vi "Entrenamiento Fuerza temp.vi"(8 "error in (no error)":errorcluster) -> (0 "error out":errorcluster)   [LabVIEW 2014]
panel:
  out "element":T1
  in  "Master":bool
  out "OK":bool
  out "error out 2":errorcluster
  in  "Puerto Serial":refnum<visa-resource-name>="COM12"
  in  "index":i32
  out "size(s)":i32
  out "Decorations[]":refnum<vi>[](array[refnum])
  out "Boolean":bool
  in  "Start":bool
  in  "Impulso":bool
  in  "Reset":bool
  in  "Back":bool
  in  "Help":bool
  in  "Slider":i32(slide) scale=0.0..100.0
  in  "Remove Button":bool
  in  "Add Button":bool
  in  "Opcional Bool":bool
  in  "Biceps Bool":bool
  in  "Pectorales Bool":bool
  in  "Trapecio Bool":bool
  in  "Dorsales Bool":bool
  in  "Lumbares Bool":bool
  in  "Abdomen Bool":bool
  in  "Gluteos Bool":bool
  in  "Isquiotibiales Bool":bool
  in  "Stop":bool
  in  "Cuadriceps Bool":bool
  # "Entrenamiento de Fuerza"
  # "Presentación"
  # "Seg"
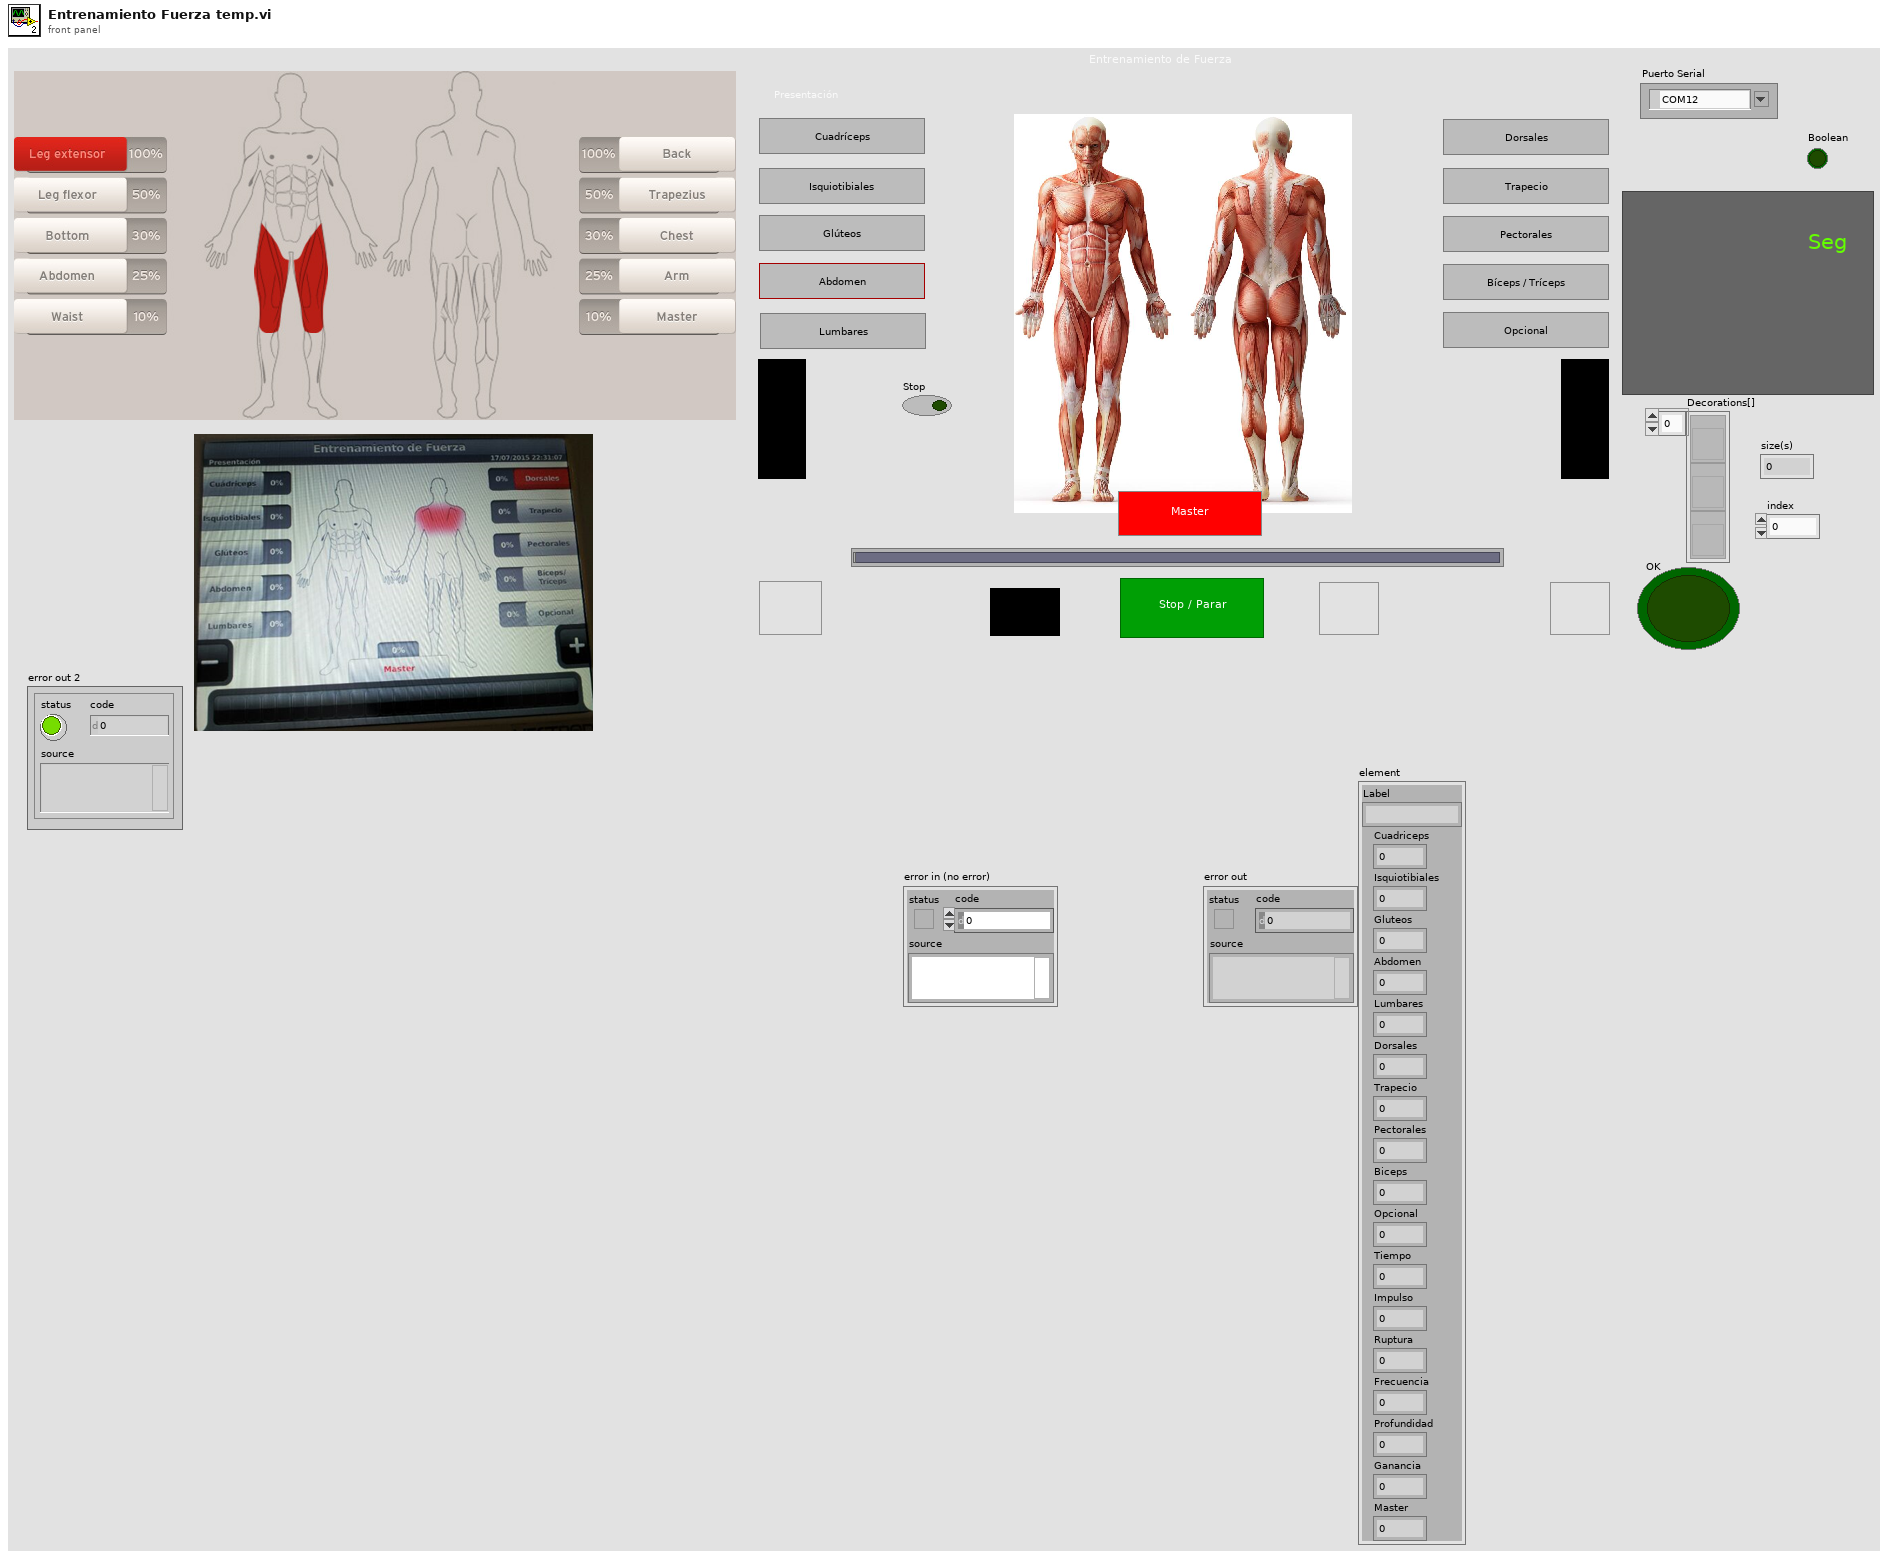
[diagram p1: front panel]
types:
  T1 = cluster{"Label":string, "Cuadriceps":i32, "Isquiotibiales":i32, "Gluteos":i32, "Abdomen":i32, "Lumbares":i32, "Dorsales":i32, "Trapecio":i32, "Pectorales":i32, "Biceps":i32, "Opcional":i32, "Tiempo":i32, "Impulso":i32, "Ruptura":i32, "Frecuencia":i32, "Profundidad":i32, "Ganancia":dbl, "Master":i32}
  T2 = cluster{"Boolean Text.Text Colors:Text Color":u32, u32}
  T3 = cluster{u32, "Boolean Text.Text Colors:Text Color":u32}
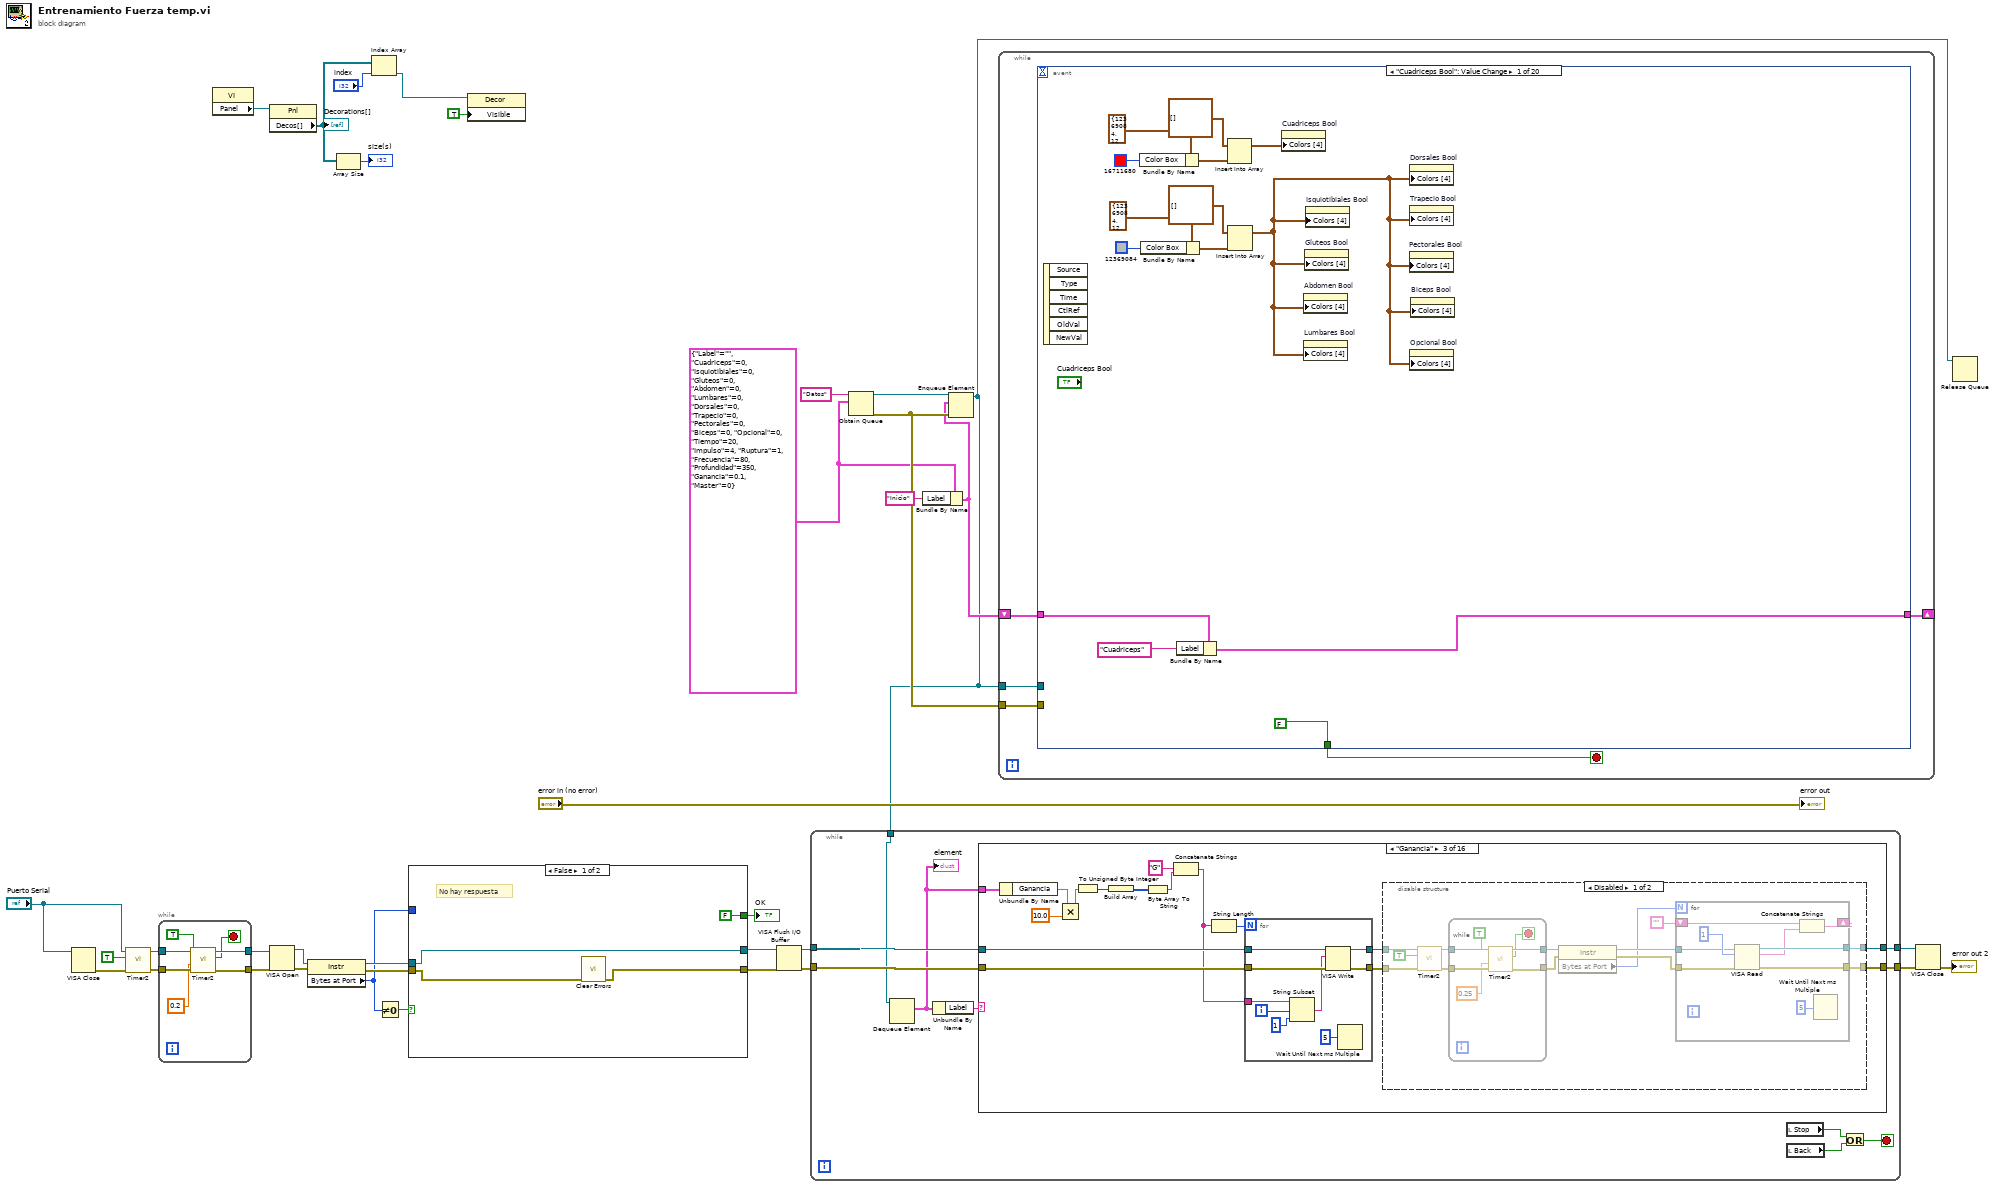
[diagram p0: block diagram]
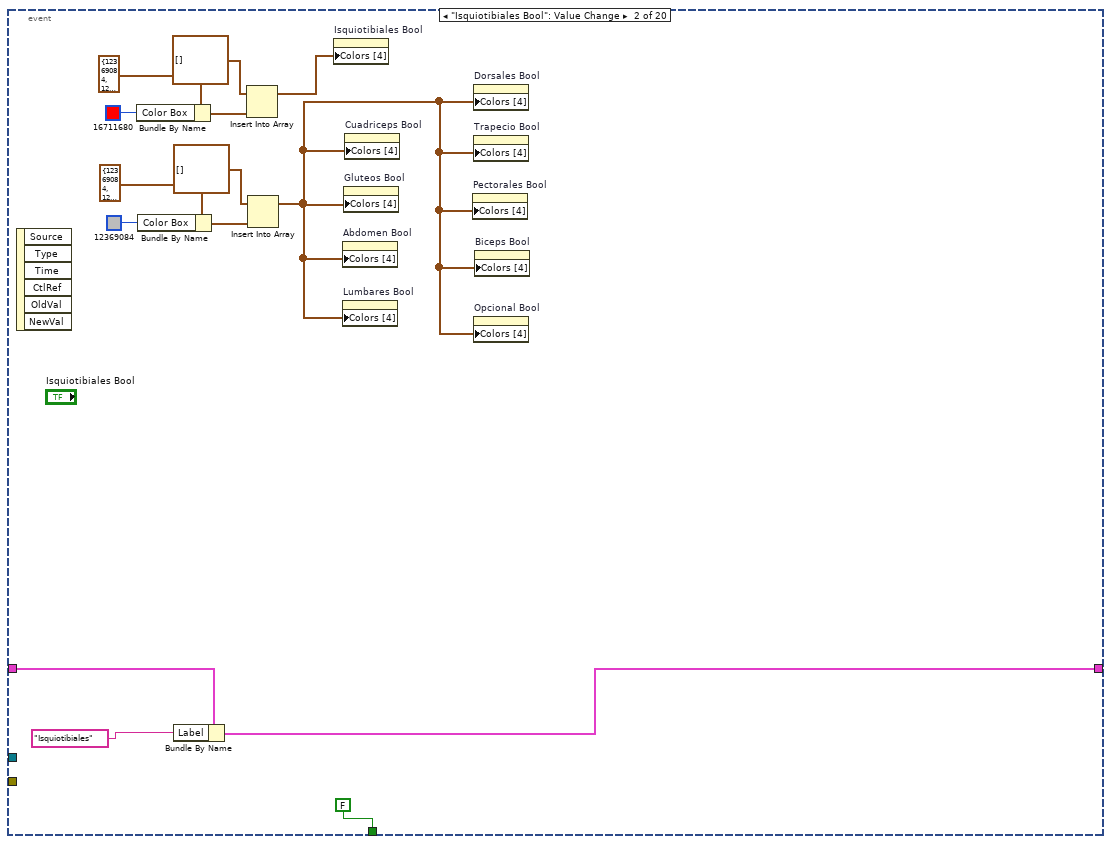
[diagram p2: hidden frame]
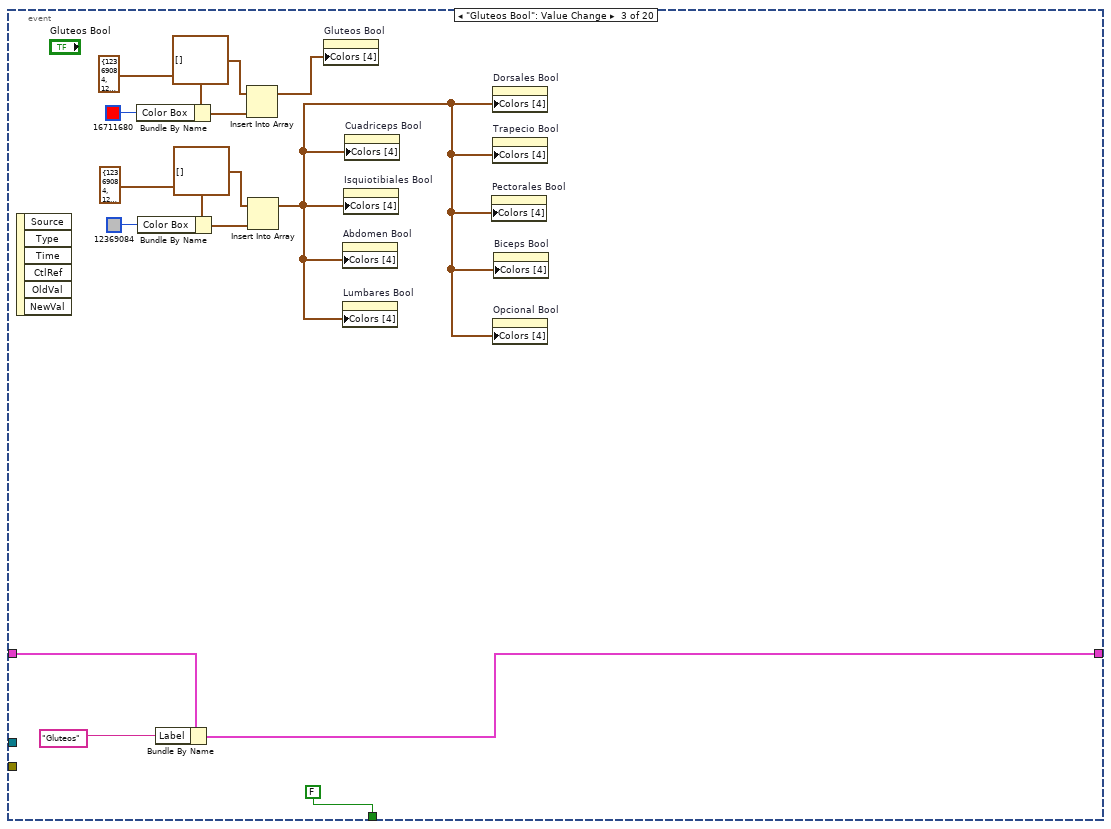
[diagram p3: hidden frame]
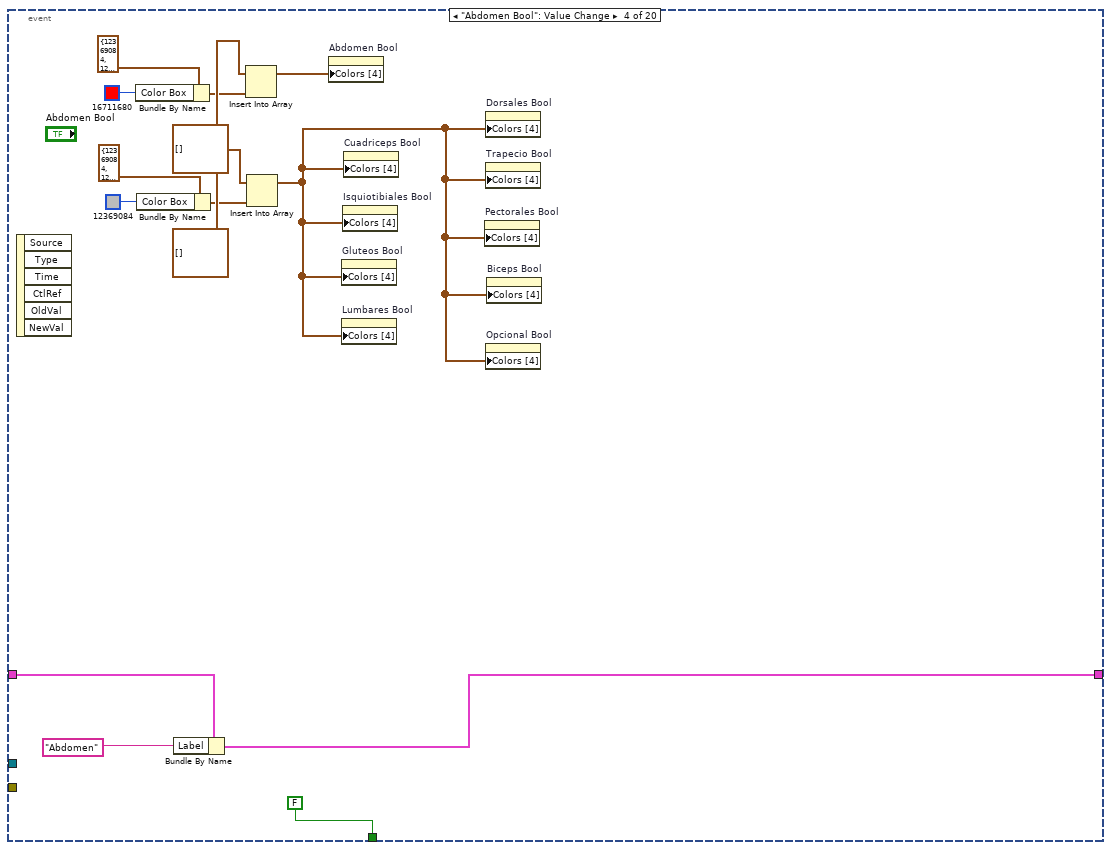
[diagram p4: hidden frame]
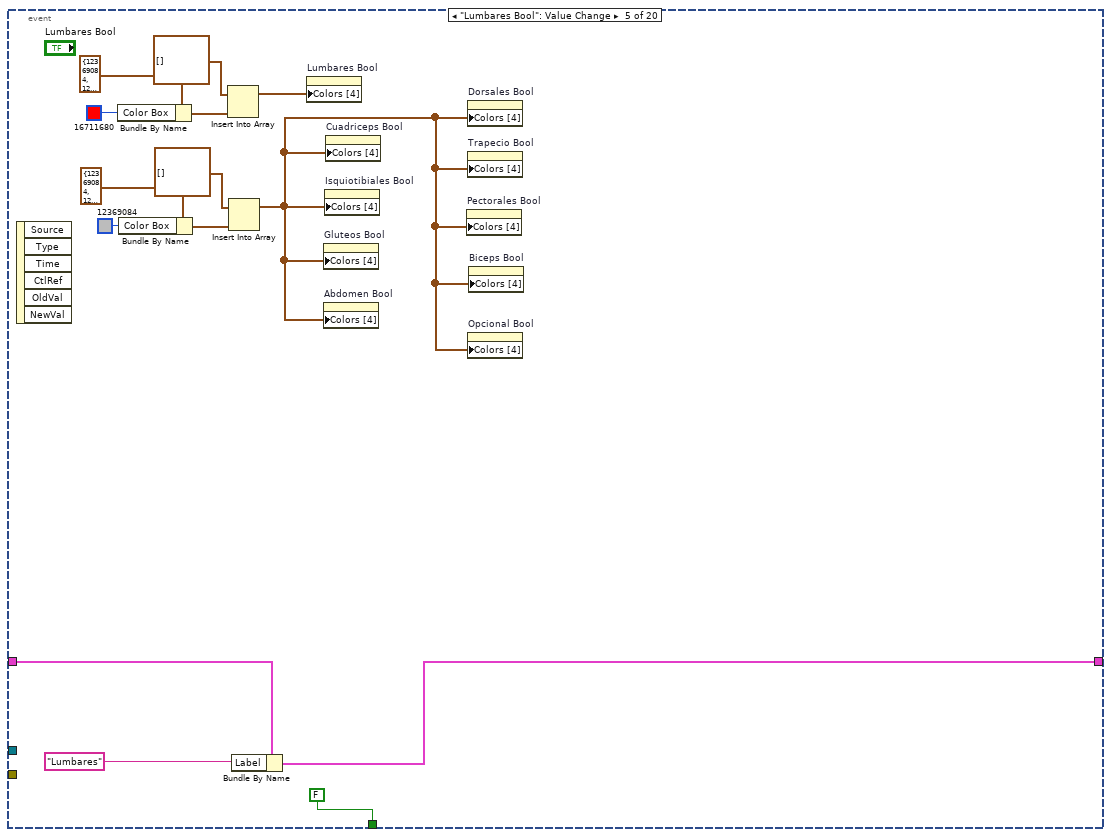
[diagram p5: hidden frame]
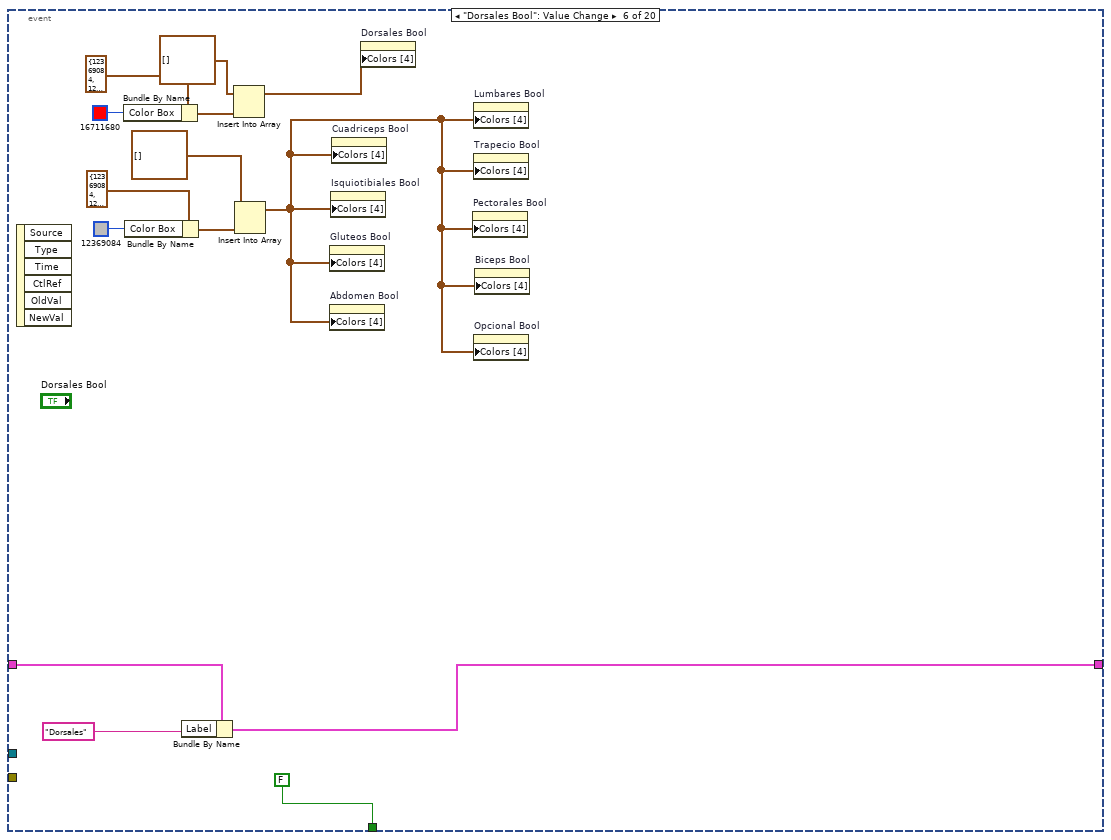
[diagram p6: hidden frame]
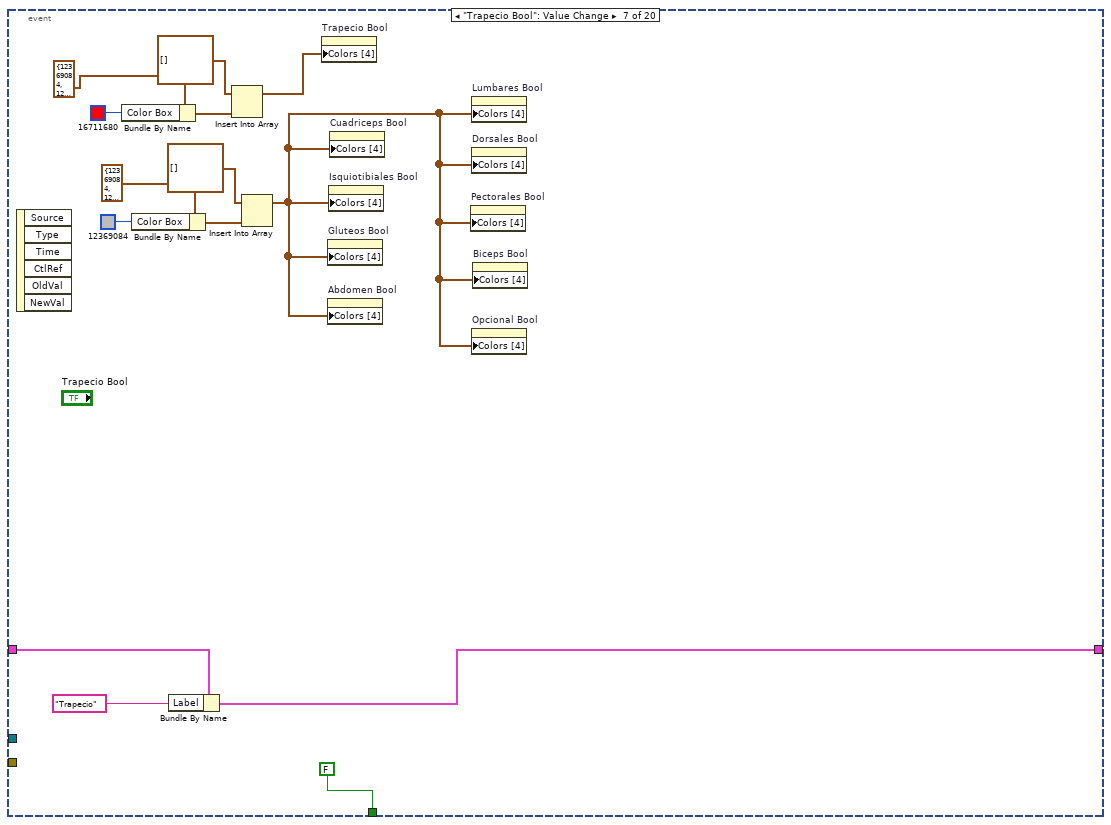
[diagram p7: hidden frame]
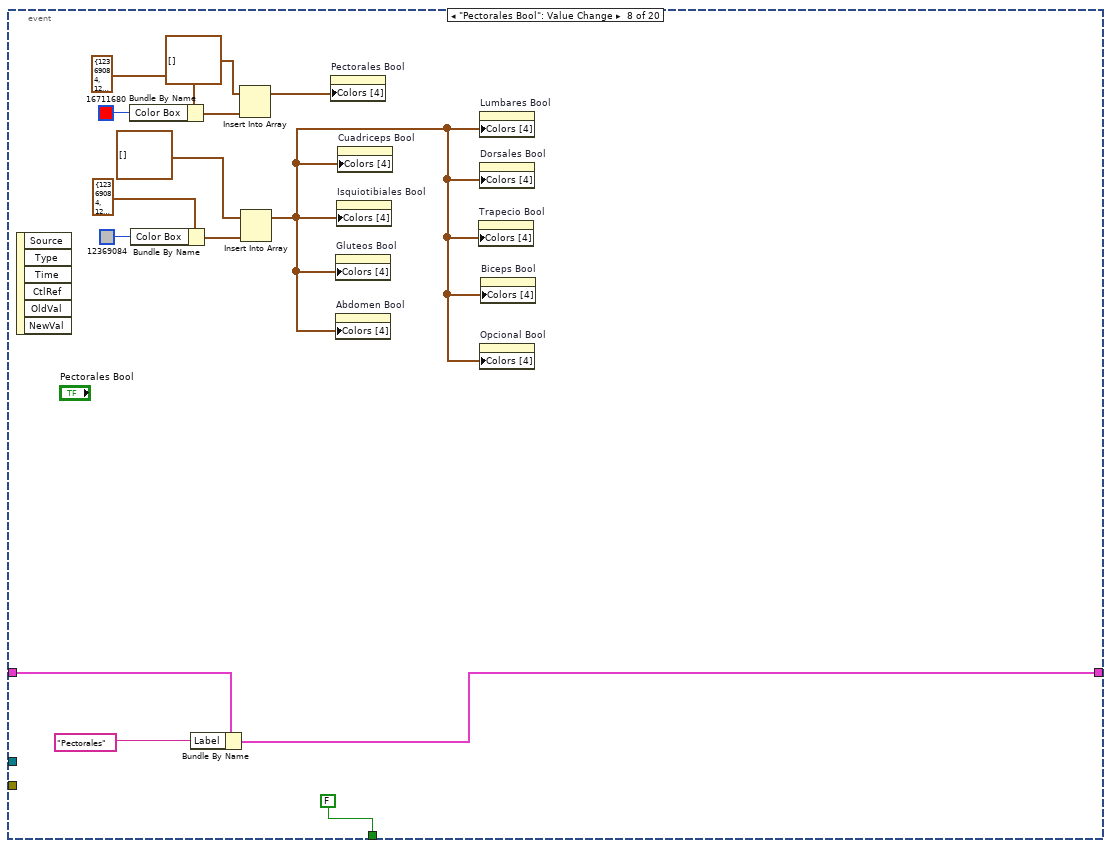
[diagram p8: hidden frame]
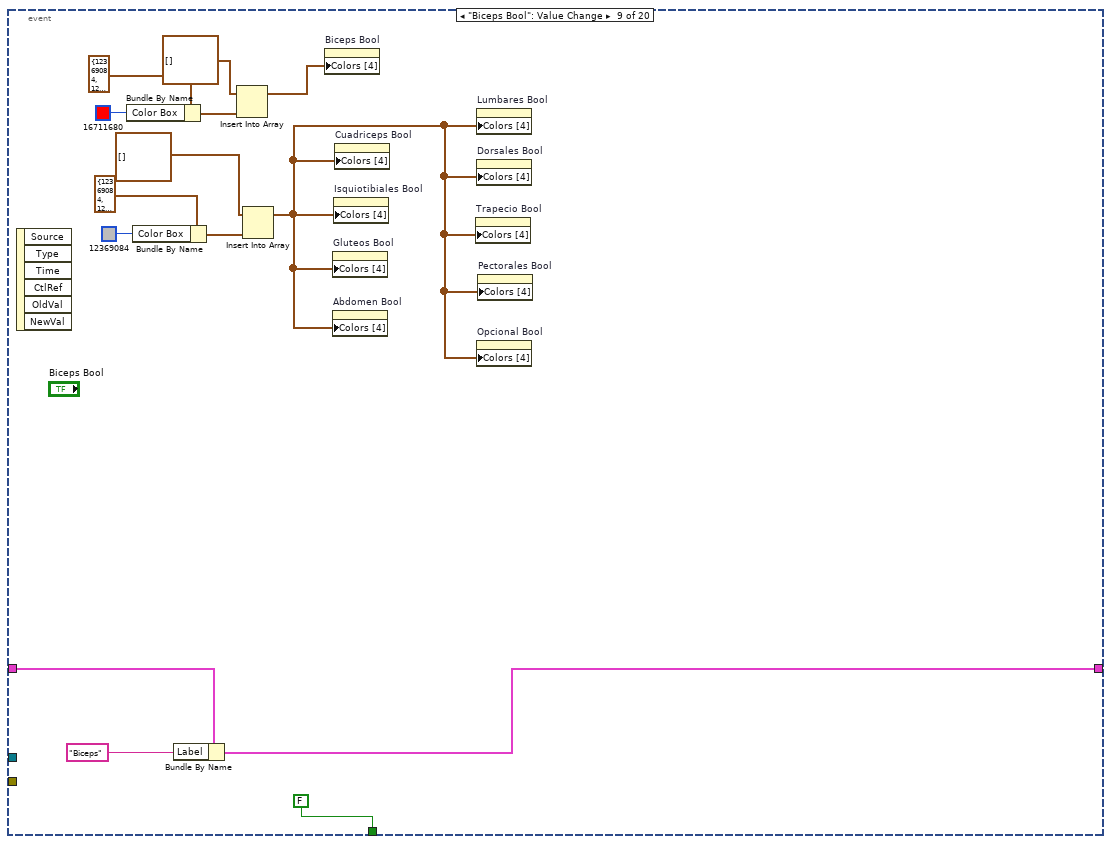
[diagram p9: hidden frame]
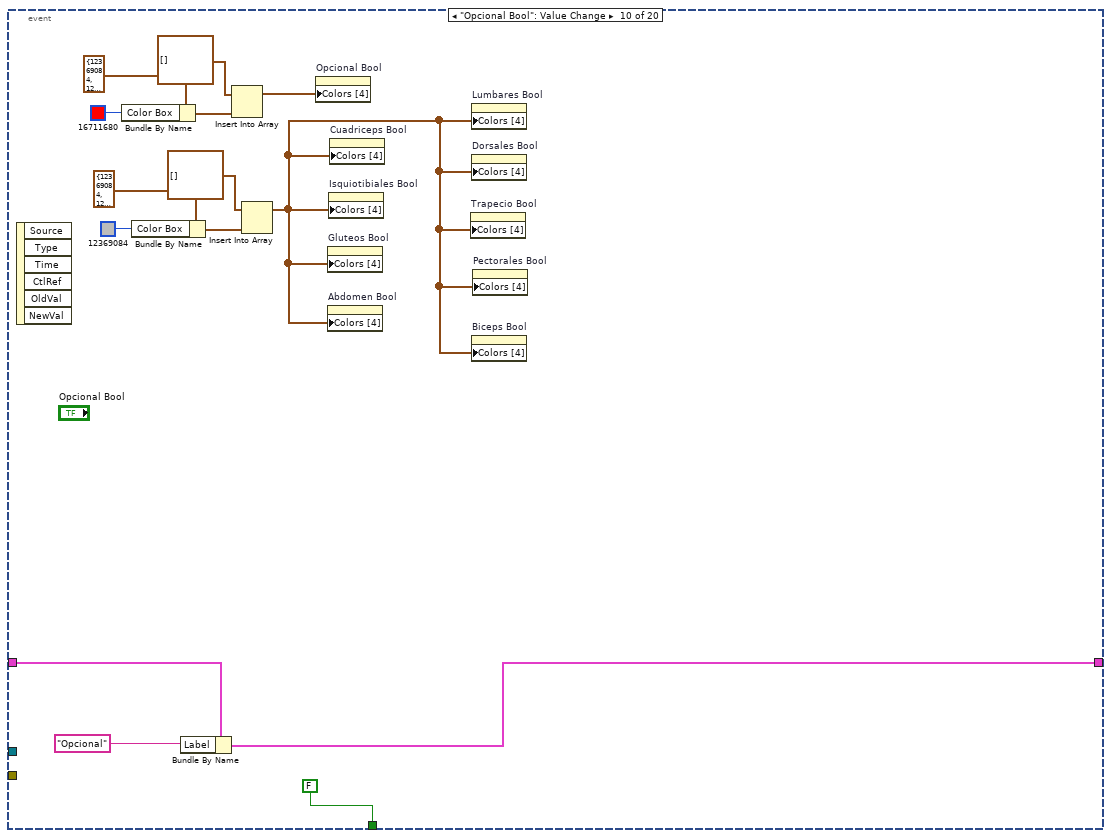
[diagram p10: hidden frame]
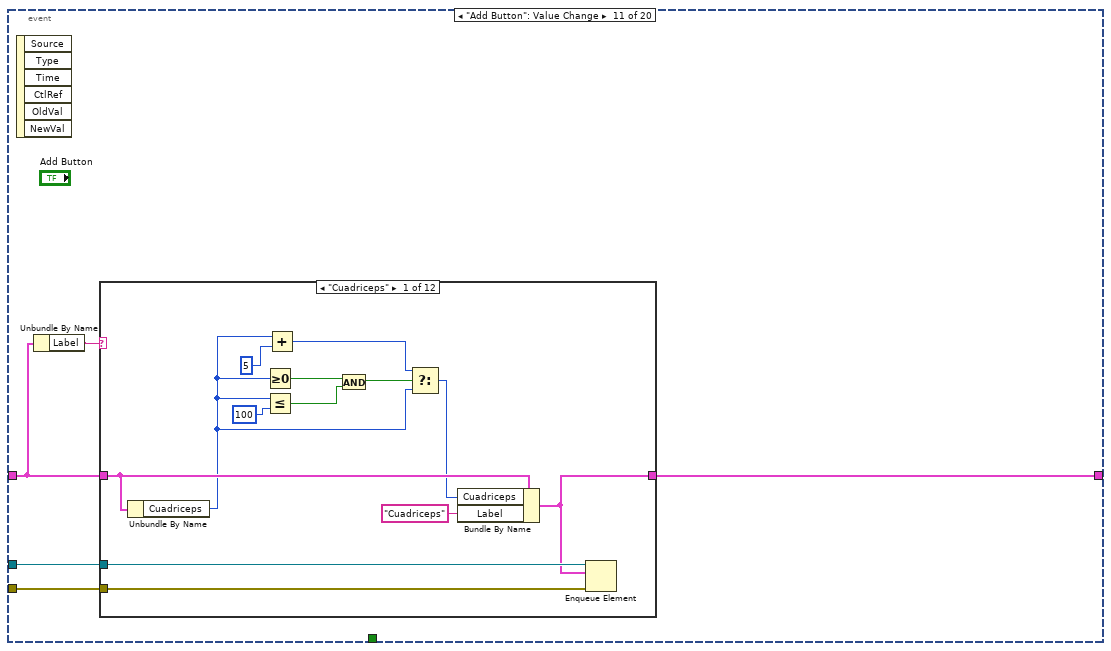
[diagram p11: hidden frame]
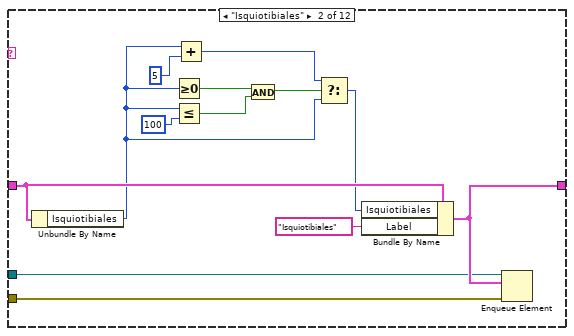
[diagram p12: hidden frame]
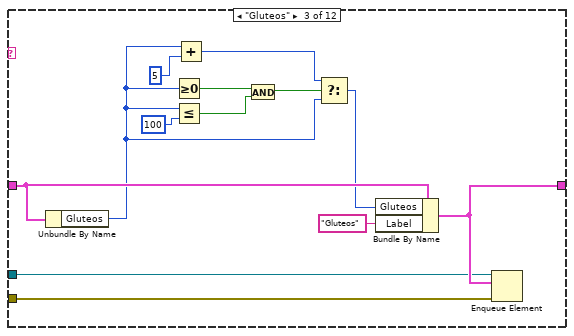
[diagram p13: hidden frame]
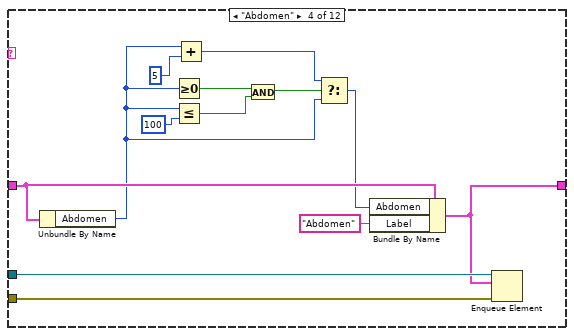
[diagram p14: hidden frame]
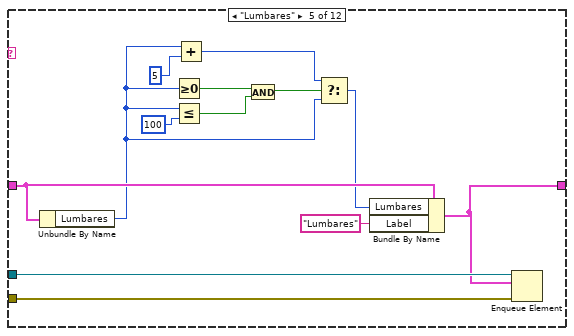
[diagram p15: hidden frame]
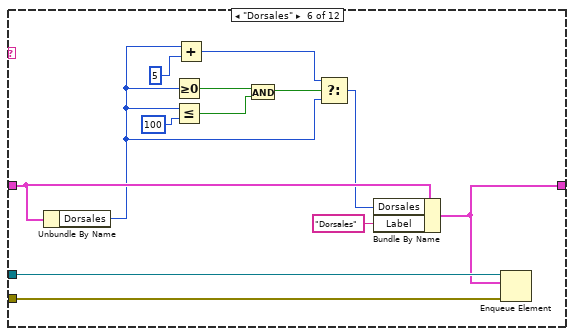
[diagram p16: hidden frame]
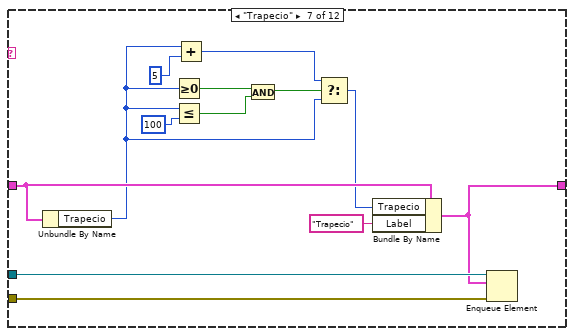
[diagram p17: hidden frame]
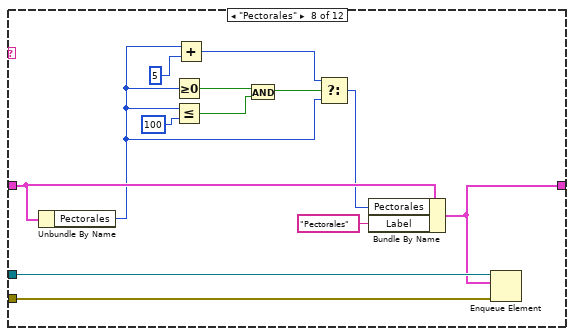
[diagram p18: hidden frame]
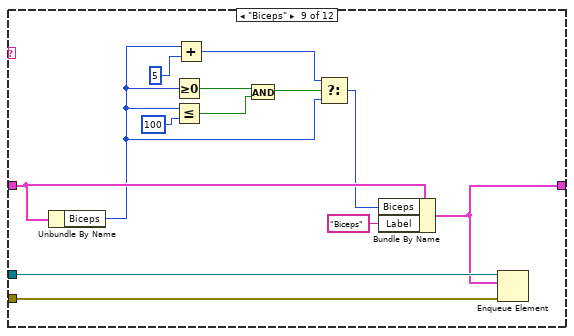
[diagram p19: hidden frame]
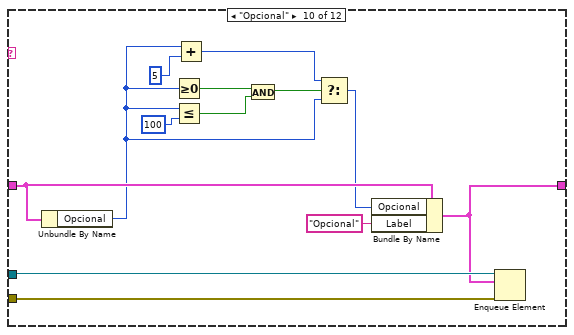
[diagram p20: hidden frame]
diagram:
  w5 = T1 {"Label"="", "Cuadriceps"=0, "Isquiotibiales"=0, "Gluteos"=0, "Abdomen"=0, "Lumbares"=0, "Dorsales"=0, "Trapecio"=0, "Pectorales"=0, "Biceps"=0, "Opcional"=0, "Tiempo"=20, "Impulso"=4, "Ruptura"=1, "Frecuencia"=80, "Profundidad"=350, "Ganancia"=0.1, "Master"=0}
  n1 = VISA Close(VISA resource name="Puerto Serial") -> (error out=w24:errorcluster)  [unwired: 1 in]
  n2 = call "Timer2.vi"("error in (no error)"=w24, "Reset"=TRUE) -> ("error out"=w23:errorcluster)  [unwired: 7 in, 2 out]
  n3 = while {
    tunnel: w23 -> [w39]
    tunnel: "Puerto Serial" -> [w40]
    tunnel: [w40] -> w25
    tunnel: [w38] -> w21
    stop <- w37 stop-if-true
    n4 = call "Timer2.vi"("error in (no error)"=w39, "Time Target (s)"=0.2, "Pause"=TRUE) -> ("error out"=w38:errorcluster, "Time has Elapsed"=w37:bool)  [unwired: 6 in, 1 out]
  }
  n5 = property class="VI"() -> ("Panel"=w33:refnum<vi>)  [unwired: 2 in, 2 out]
  n6 = property class="Pnl"(reference=w33) -> ("Decos[]"=w30:refnum<vi>[])  [unwired: 1 in, 2 out]
  "Decorations[]" <- w30
  n7 = VISA Open(error in (no error)=w21, VISA resource name=w25) -> (VISA resource name=w10:refnum<visa-resource-name>, error out=w14:errorcluster)  [unwired: 3 in]
  n8 = property class="Instr"(reference=w10, error in=w14) -> (reference out=w19:refnum<visa-resource-name>, error out=w20:errorcluster, "Bytes at Port"=w17:u32)
  n9 = Array Size(array=w30) -> (size(s)=→"size(s)":i32)
  n10 = Index Array(array=w30, index="index") -> (element=w29:refnum<vi>)
  n11 = Not Equal To 0?(x=w17) -> (x != 0?=w18:bool)
  n12 = case shown="False" w18 {
    tunnel: w20 -> [w42 w52]
    tunnel: w19 -> [w44 w51]
    tunnel: w17 -> [_ w50]
    tunnel: [w44 w48] -> w15
    tunnel: [w41 w47] -> w16
    tunnel: [FALSE w46] -> w11
    frame False {
      # "No hay respuesta"
      n13 = call <vilib>:"Clear Errors.vi"("error in (no error)"=w42) -> ("error out"=w41:errorcluster)  [unwired: 5 in, 1 out]
    }
    frame True {
      # "Recibe Datos de Respuesta"
      n14 = for {
        N: w50 -> [_]
        tunnel: w52 -> [w61]
        tunnel: w51 -> [w60]
        shift-right: [w55] -> w45
        shift-left: "" -> [w59]
        tunnel: [w58] -> w47
        tunnel: [w57] -> w48
        n15 = VISA Read(VISA resource name=w60, byte count=u32 1, error in (no error)=w61) -> (VISA resource name out=w57:refnum<visa-resource-name>, read buffer=w54:string, error out=w58:errorcluster)  [unwired: 1 out]
        n16 = Concatenate Strings(w59, w54) -> (w55:string)
        n17 = Wait Until Next ms Multiple(millisecond multiple=u32 1) -> ()  [unwired: 1 out]
      }
      n18 = Equal?(x=w45, y="OK") -> (x = y?=w46:bool)
    }
  }
  "OK" <- w11
  n19 = property class="Decor"(reference=w29, "Visible"=TRUE) -> ()  [unwired: 1 in, 2 out]
  n20 = VISA Flush I/O Buffer(VISA resource name=w15, error in (no error)=w16) -> (VISA resource name out=w12:refnum<visa-resource-name>, error out=w13:errorcluster)  [unwired: 1 in]
  n21 = Obtain Queue(name (unnamed)="Datos", element data type=w5) -> (queue out=w6:refnum<queue>, error out=w7:errorcluster)  [unwired: 3 in, 1 out]
  n22 = Bundle By Name(cluster=w5, "Label"="Inicio") -> (w3:T1)
  n23 = Enqueue Element(queue=w6, element=w3, error in (no error)=w7) -> (queue out=w2:refnum<queue>)  [unwired: 1 in, 2 out]
  n24 = while {
    tunnel: w12 -> [w72]
    tunnel: [w69] -> w8
    tunnel: w13 -> [w71]
    tunnel: [w70] -> w9
    tunnel: w2 -> [w63]
    stop <- w65 stop-if-true
    n25 = Dequeue Element(queue=w63) -> (element=w64:T1)  [unwired: 2 in, 3 out]
    "element" <- w64
    n26 = Unbundle By Name(w64) -> ("Label"=w68:string)
    n27 = case shown="\"Ganancia\"" w68 {
      tunnel: w72 -> [w73 w88 w142 w196 w248 w290 w351 w403 w455 w507 w559 w611 w663 w715 w767 w819]
      tunnel: w71 -> [w74 w87 w141 w195 w247 w289 w350 w402 w454 w506 w558 w610 w662 w714 w766 w818]
      tunnel: [w74 w86 w140 w194 w246 w292 w349 w401 w453 w505 w557 w609 w661 w713 w765 w817] -> w70
      tunnel: [w73 w85 w139 w193 w245 w291 w348 w400 w452 w504 w556 w608 w660 w712 w764 w816] -> w69
      tunnel: w64 -> [_ w77 w132 w186 w235 w307 w340 w392 w444 w496 w548 w600 w652 w704 w756 w808]
      frame "Inicio", Default {
      }
      frame "Frecuencia" {
        n28 = Unbundle By Name(w77) -> ("Frecuencia"=w78:i32)
        n29 = To Unsigned Byte Integer(number=w78) -> (unsigned 8bit integer=w76:u8)
        n30 = Build Array(w76) -> (w75:u8[])
        n31 = Byte Array To String(unsigned byte array=w75) -> (string=w80:string)
        n32 = Concatenate Strings("F", w80) -> (w79:string)
        n33 = String Length(string=w79) -> (length=w84:i32)
        n34 = for {
          N: w84 -> [_]
          tunnel: w87 -> [w126]
          tunnel: w88 -> [w125]
          tunnel: w79 -> [w122]
          tunnel: [w119] -> w82
          tunnel: [w118] -> w83
          i -> [w120]
          n35 = String Subset(string=w122, offset (0)=w120, length (rest)=1 ("length (rest)")) -> (substring=w123:string)
          n36 = VISA Write(VISA resource name=w125, write buffer=w123, error in (no error)=w126) -> (VISA resource name out=w118:refnum<visa-resource-name>, error out=w119:errorcluster)  [unwired: 1 out]
          n37 = Wait Until Next ms Multiple(millisecond multiple=u32 5) -> ()  [unwired: 1 out]
        }
        n38 = disable-structure shown="Disabled" {
          disable-tunnel: [w100 w116] -> w86
          disable-tunnel: [w99 w117] -> w85
          disable-tunnel: w83 -> [w94 w117]
          disable-tunnel: w82 -> [w90 w116]
          frame Disabled {
            n39 = call "Timer2.vi"("error in (no error)"=w90, "Reset"=TRUE) -> ("error out"=w89:errorcluster)  [unwired: 7 in, 2 out]
            n40 = while {
              tunnel: w94 -> [w106]
              tunnel: [w106] -> w93
              tunnel: [w104] -> w92
              tunnel: w89 -> [w105]
              stop <- w103 stop-if-true
              n41 = call "Timer2.vi"("error in (no error)"=w105, "Time Target (s)"=0.25, "Pause"=TRUE) -> ("error out"=w104:errorcluster, "Time has Elapsed"=w103:bool)  [unwired: 6 in, 1 out]
            }
            n42 = property class="Instr"(reference=w93, error in=w92) -> (reference out=w97:refnum<visa-resource-name>, error out=w96:errorcluster, "Bytes at Port"=w95:u32)
            n43 = for {
              N: w95 -> [_]
              tunnel: w96 -> [w114]
              tunnel: w97 -> [w113]
              shift-right: [w108] -> _
              shift-left: "" -> [w112]
              tunnel: [w111] -> w100
              tunnel: [w110] -> w99
              n44 = VISA Read(VISA resource name=w113, byte count=u32 1, error in (no error)=w114) -> (VISA resource name out=w110:refnum<visa-resource-name>, read buffer=w107:string, error out=w111:errorcluster)  [unwired: 1 out]
              n45 = Concatenate Strings(w112, w107) -> (w108:string)
              n46 = Wait Until Next ms Multiple(millisecond multiple=u32 5) -> ()  [unwired: 1 out]
            }
          }
          frame Enabled {
          }
        }
      }
      frame "Ganancia" {
        n47 = Unbundle By Name(w132) -> ("Ganancia"=w128:dbl)
        n48 = Multiply(x=w128, y=10.0) -> (x*y=w129:dbl)
        n49 = To Unsigned Byte Integer(number=w129) -> (unsigned 8bit integer=w131:u8)
        n50 = Build Array(w131) -> (w130:u8[])
        n51 = Byte Array To String(unsigned byte array=w130) -> (string=w134:string)
        n52 = Concatenate Strings("G", w134) -> (w133:string)
        n53 = String Length(string=w133) -> (length=w138:i32)
        n54 = for {
          N: w138 -> [_]
          tunnel: w141 -> [w180]
          tunnel: w142 -> [w179]
          tunnel: w133 -> [w176]
          tunnel: [w173] -> w136
          tunnel: [w172] -> w137
          i -> [w174]
          n55 = String Subset(string=w176, offset (0)=w174, length (rest)=1 ("length (rest)")) -> (substring=w177:string)
          n56 = VISA Write(VISA resource name=w179, write buffer=w177, error in (no error)=w180) -> (VISA resource name out=w172:refnum<visa-resource-name>, error out=w173:errorcluster)  [unwired: 1 out]
          n57 = Wait Until Next ms Multiple(millisecond multiple=u32 5) -> ()  [unwired: 1 out]
        }
        n58 = disable-structure shown="Disabled" {
          disable-tunnel: [w154 w170] -> w140
          disable-tunnel: [w153 w171] -> w139
          disable-tunnel: w137 -> [w148 w171]
          disable-tunnel: w136 -> [w144 w170]
          frame Disabled {
            n59 = call "Timer2.vi"("error in (no error)"=w144, "Reset"=TRUE) -> ("error out"=w143:errorcluster)  [unwired: 7 in, 2 out]
            n60 = while {
              tunnel: w148 -> [w160]
              tunnel: [w160] -> w147
              tunnel: [w158] -> w146
              tunnel: w143 -> [w159]
              stop <- w157 stop-if-true
              n61 = call "Timer2.vi"("error in (no error)"=w159, "Time Target (s)"=0.25, "Pause"=TRUE) -> ("error out"=w158:errorcluster, "Time has Elapsed"=w157:bool)  [unwired: 6 in, 1 out]
            }
            n62 = property class="Instr"(reference=w147, error in=w146) -> (reference out=w151:refnum<visa-resource-name>, error out=w150:errorcluster, "Bytes at Port"=w149:u32)
            n63 = for {
              N: w149 -> [_]
              tunnel: w150 -> [w168]
              tunnel: w151 -> [w167]
              shift-right: [w162] -> _
              shift-left: "" -> [w166]
              tunnel: [w165] -> w154
              tunnel: [w164] -> w153
              n64 = VISA Read(VISA resource name=w167, byte count=u32 1, error in (no error)=w168) -> (VISA resource name out=w164:refnum<visa-resource-name>, read buffer=w161:string, error out=w165:errorcluster)  [unwired: 1 out]
              n65 = Concatenate Strings(w166, w161) -> (w162:string)
              n66 = Wait Until Next ms Multiple(millisecond multiple=u32 5) -> ()  [unwired: 1 out]
            }
          }
          frame Enabled {
          }
        }
      }
      frame "Impulso" {
        n67 = Unbundle By Name(w186) -> ("Profundidad"=w183:i32)
        n68 = To Unsigned Word Integer(number=w183) -> (unsigned 16bit integer=w182:u16)
        n69 = Split Number(x=w182) -> (hi(x)=w185:u8, lo(x)=w184:u8)
        n70 = Build Array(w185, w184) -> (w181:u8[])
        n71 = Byte Array To String(unsigned byte array=w181) -> (string=w188:string)
        n72 = Concatenate Strings("P", w188) -> (w187:string)
        n73 = String Length(string=w187) -> (length=w192:i32)
        n74 = for {
          N: w192 -> [_]
          tunnel: w195 -> [w234]
          tunnel: w196 -> [w233]
          tunnel: w187 -> [w230]
          tunnel: [w227] -> w190
          tunnel: [w226] -> w191
          i -> [w228]
          n75 = String Subset(string=w230, offset (0)=w228, length (rest)=1 ("length (rest)")) -> (substring=w231:string)
          n76 = VISA Write(VISA resource name=w233, write buffer=w231, error in (no error)=w234) -> (VISA resource name out=w226:refnum<visa-resource-name>, error out=w227:errorcluster)  [unwired: 1 out]
          n77 = Wait Until Next ms Multiple(millisecond multiple=u32 5) -> ()  [unwired: 1 out]
        }
        n78 = disable-structure shown="Disabled" {
          disable-tunnel: [w208 w224] -> w194
          disable-tunnel: [w207 w225] -> w193
          disable-tunnel: w191 -> [w202 w225]
          disable-tunnel: w190 -> [w198 w224]
          frame Disabled {
            n79 = call "Timer2.vi"("error in (no error)"=w198, "Reset"=TRUE) -> ("error out"=w197:errorcluster)  [unwired: 7 in, 2 out]
            n80 = while {
              tunnel: w202 -> [w214]
              tunnel: [w214] -> w201
              tunnel: [w212] -> w200
              tunnel: w197 -> [w213]
              stop <- w211 stop-if-true
              n81 = call "Timer2.vi"("error in (no error)"=w213, "Time Target (s)"=0.25, "Pause"=TRUE) -> ("error out"=w212:errorcluster, "Time has Elapsed"=w211:bool)  [unwired: 6 in, 1 out]
            }
            n82 = property class="Instr"(reference=w201, error in=w200) -> (reference out=w205:refnum<visa-resource-name>, error out=w204:errorcluster, "Bytes at Port"=w203:u32)
            n83 = for {
              N: w203 -> [_]
              tunnel: w204 -> [w222]
              tunnel: w205 -> [w221]
              shift-right: [w216] -> _
              shift-left: "" -> [w220]
              tunnel: [w219] -> w208
              tunnel: [w218] -> w207
              n84 = VISA Read(VISA resource name=w221, byte count=u32 1, error in (no error)=w222) -> (VISA resource name out=w218:refnum<visa-resource-name>, read buffer=w215:string, error out=w219:errorcluster)  [unwired: 1 out]
              n85 = Concatenate Strings(w220, w215) -> (w216:string)
              n86 = Wait Until Next ms Multiple(millisecond multiple=u32 5) -> ()  [unwired: 1 out]
            }
          }
          frame Enabled {
          }
        }
      }
      frame "Master" {
        n87 = Unbundle By Name(w235) -> ("Master"=w238:i32)
        n88 = To Unsigned Byte Integer(number=w238) -> (unsigned 8bit integer=w237:u8)
        n89 = Build Array(w237) -> (w236:u8[])
        n90 = Byte Array To String(unsigned byte array=w236) -> (string=w240:string)
        n91 = Concatenate Strings("M", w240) -> (w239:string)
        n92 = String Length(string=w239) -> (length=w244:i32)
        n93 = for {
          N: w244 -> [_]
          tunnel: w247 -> [w286]
          tunnel: w248 -> [w285]
          tunnel: w239 -> [w282]
          tunnel: [w279] -> w242
          tunnel: [w278] -> w243
          i -> [w280]
          n94 = String Subset(string=w282, offset (0)=w280, length (rest)=1 ("length (rest)")) -> (substring=w283:string)
          n95 = VISA Write(VISA resource name=w285, write buffer=w283, error in (no error)=w286) -> (VISA resource name out=w278:refnum<visa-resource-name>, error out=w279:errorcluster)  [unwired: 1 out]
          n96 = Wait Until Next ms Multiple(millisecond multiple=u32 5) -> ()  [unwired: 1 out]
        }
        n97 = disable-structure shown="Disabled" {
          disable-tunnel: [w260 w276] -> w246
          disable-tunnel: [w259 w277] -> w245
          disable-tunnel: w243 -> [w254 w277]
          disable-tunnel: w242 -> [w250 w276]
          frame Disabled {
            n98 = call "Timer2.vi"("error in (no error)"=w250, "Reset"=TRUE) -> ("error out"=w249:errorcluster)  [unwired: 7 in, 2 out]
            n99 = while {
              tunnel: w254 -> [w266]
              tunnel: [w266] -> w253
              tunnel: [w264] -> w252
              tunnel: w249 -> [w265]
              stop <- w263 stop-if-true
              n100 = call "Timer2.vi"("error in (no error)"=w265, "Time Target (s)"=0.25, "Pause"=TRUE) -> ("error out"=w264:errorcluster, "Time has Elapsed"=w263:bool)  [unwired: 6 in, 1 out]
            }
            n101 = property class="Instr"(reference=w253, error in=w252) -> (reference out=w257:refnum<visa-resource-name>, error out=w256:errorcluster, "Bytes at Port"=w255:u32)
            n102 = for {
              N: w255 -> [_]
              tunnel: w256 -> [w274]
              tunnel: w257 -> [w273]
              shift-right: [w268] -> _
              shift-left: "" -> [w272]
              tunnel: [w271] -> w260
              tunnel: [w270] -> w259
              n103 = VISA Read(VISA resource name=w273, byte count=u32 1, error in (no error)=w274) -> (VISA resource name out=w270:refnum<visa-resource-name>, read buffer=w267:string, error out=w271:errorcluster)  [unwired: 1 out]
              n104 = Concatenate Strings(w272, w267) -> (w268:string)
              n105 = Wait Until Next ms Multiple(millisecond multiple=u32 5) -> ()  [unwired: 1 out]
            }
          }
          frame Enabled {
          }
        }
      }
      frame "Encender" {
        w297 = "A"
        w303 = "E"
        n106 = Unbundle By Name(w307) -> ("Impulso"=w288:i32, "Ruptura"=w287:i32)
        n107 = String Length(string=w303) -> (length=w306:i32)
        n108 = for {
          N: w306 -> [_]
          tunnel: w289 -> [w337]
          tunnel: w290 -> [w336]
          tunnel: w303 -> [w333]
          tunnel: [w330] -> w304
          tunnel: [w329] -> w305
          i -> [w331]
          n109 = String Subset(string=w333, offset (0)=w331, length (rest)=1 ("length (rest)")) -> (substring=w334:string)
          n110 = VISA Write(VISA resource name=w336, write buffer=w334, error in (no error)=w337) -> (VISA resource name out=w329:refnum<visa-resource-name>, error out=w330:errorcluster)  [unwired: 1 out]
          n111 = Wait Until Next ms Multiple(millisecond multiple=u32 5) -> ()  [unwired: 1 out]
        }
        n112 = call "Timer2.vi"("error in (no error)"=w304, "Reset"=TRUE) -> ("error out"=w301:errorcluster)  [unwired: 7 in, 2 out]
        n113 = while {
          tunnel: w305 -> [w328]
          tunnel: [w328] -> w294
          tunnel: [w326] -> w293
          tunnel: w301 -> [w327]
          tunnel: w288 -> [w323]
          stop <- w325 stop-if-true
          n114 = call "Timer2.vi"("error in (no error)"=w327, "Time Target (s)"=w323, "Pause"=TRUE) -> ("error out"=w326:errorcluster, "Time has Elapsed"=w325:bool)  [unwired: 6 in, 1 out]
        }
        n115 = String Length(string=w297) -> (length=w300:i32)
        n116 = for {
          N: w300 -> [_]
          tunnel: w293 -> [w322]
          tunnel: w294 -> [w321]
          tunnel: w297 -> [w318]
          tunnel: [w315] -> w298
          tunnel: [w314] -> w299
          i -> [w316]
          n117 = String Subset(string=w318, offset (0)=w316, length (rest)=1 ("length (rest)")) -> (substring=w319:string)
          n118 = VISA Write(VISA resource name=w321, write buffer=w319, error in (no error)=w322) -> (VISA resource name out=w314:refnum<visa-resource-name>, error out=w315:errorcluster)  [unwired: 1 out]
          n119 = Wait Until Next ms Multiple(millisecond multiple=u32 5) -> ()  [unwired: 1 out]
        }
        n120 = call "Timer2.vi"("error in (no error)"=w298, "Reset"=TRUE) -> ("error out"=w295:errorcluster)  [unwired: 7 in, 2 out]
        n121 = while {
          tunnel: w299 -> [w313]
          tunnel: [w313] -> w291
          tunnel: [w311] -> w292
          tunnel: w295 -> [w312]
          tunnel: w287 -> [w308]
          stop <- w310 stop-if-true
          n122 = call "Timer2.vi"("error in (no error)"=w312, "Time Target (s)"=w308, "Pause"=TRUE) -> ("error out"=w311:errorcluster, "Time has Elapsed"=w310:bool)  [unwired: 6 in, 1 out]
        }
      }
      frame "Cuadriceps" {
        n123 = Unbundle By Name(w340) -> ("Cuadriceps"=w338:i32)
        n124 = To Unsigned Byte Integer(number=w338) -> (unsigned 8bit integer=w339:u8)
        n125 = Build Array(w339) -> (w344:u8[])
        n126 = Byte Array To String(unsigned byte array=w344) -> (string=w342:string)
        n127 = Concatenate Strings("1", w342) -> (w341:string)
        n128 = String Length(string=w341) -> (length=w347:i32)
        n129 = for {
          N: w347 -> [_]
          tunnel: w350 -> [w389]
          tunnel: w351 -> [w388]
          tunnel: w341 -> [w385]
          tunnel: [w382] -> w345
          tunnel: [w381] -> w346
          i -> [w383]
          n130 = String Subset(string=w385, offset (0)=w383, length (rest)=1 ("length (rest)")) -> (substring=w386:string)
          n131 = VISA Write(VISA resource name=w388, write buffer=w386, error in (no error)=w389) -> (VISA resource name out=w381:refnum<visa-resource-name>, error out=w382:errorcluster)  [unwired: 1 out]
          n132 = Wait Until Next ms Multiple(millisecond multiple=u32 5) -> ()  [unwired: 1 out]
        }
        n133 = disable-structure shown="Disabled" {
          disable-tunnel: [w363 w379] -> w349
          disable-tunnel: [w362 w380] -> w348
          disable-tunnel: w346 -> [w357 w380]
          disable-tunnel: w345 -> [w353 w379]
          frame Disabled {
            n134 = call "Timer2.vi"("error in (no error)"=w353, "Reset"=TRUE) -> ("error out"=w352:errorcluster)  [unwired: 7 in, 2 out]
            n135 = while {
              tunnel: w357 -> [w369]
              tunnel: [w369] -> w356
              tunnel: [w367] -> w355
              tunnel: w352 -> [w368]
              stop <- w366 stop-if-true
              n136 = call "Timer2.vi"("error in (no error)"=w368, "Time Target (s)"=0.25, "Pause"=TRUE) -> ("error out"=w367:errorcluster, "Time has Elapsed"=w366:bool)  [unwired: 6 in, 1 out]
            }
            n137 = property class="Instr"(reference=w356, error in=w355) -> (reference out=w360:refnum<visa-resource-name>, error out=w359:errorcluster, "Bytes at Port"=w358:u32)
            n138 = for {
              N: w358 -> [_]
              tunnel: w359 -> [w377]
              tunnel: w360 -> [w376]
              shift-right: [w371] -> _
              shift-left: "" -> [w375]
              tunnel: [w374] -> w363
              tunnel: [w373] -> w362
              n139 = VISA Read(VISA resource name=w376, byte count=u32 1, error in (no error)=w377) -> (VISA resource name out=w373:refnum<visa-resource-name>, read buffer=w370:string, error out=w374:errorcluster)  [unwired: 1 out]
              n140 = Concatenate Strings(w375, w370) -> (w371:string)
              n141 = Wait Until Next ms Multiple(millisecond multiple=u32 5) -> ()  [unwired: 1 out]
            }
          }
          frame Enabled {
          }
        }
      }
      frame "Isquiotibiales" {
        n142 = Unbundle By Name(w392) -> ("Isquiotibiales"=w390:i32)
        n143 = To Unsigned Byte Integer(number=w390) -> (unsigned 8bit integer=w391:u8)
        n144 = Build Array(w391) -> (w396:u8[])
        n145 = Byte Array To String(unsigned byte array=w396) -> (string=w394:string)
        n146 = Concatenate Strings("2", w394) -> (w393:string)
        n147 = String Length(string=w393) -> (length=w399:i32)
        n148 = for {
          N: w399 -> [_]
          tunnel: w402 -> [w441]
          tunnel: w403 -> [w440]
          tunnel: w393 -> [w437]
          tunnel: [w434] -> w397
          tunnel: [w433] -> w398
          i -> [w435]
          n149 = String Subset(string=w437, offset (0)=w435, length (rest)=1 ("length (rest)")) -> (substring=w438:string)
          n150 = VISA Write(VISA resource name=w440, write buffer=w438, error in (no error)=w441) -> (VISA resource name out=w433:refnum<visa-resource-name>, error out=w434:errorcluster)  [unwired: 1 out]
          n151 = Wait Until Next ms Multiple(millisecond multiple=u32 5) -> ()  [unwired: 1 out]
        }
        n152 = disable-structure shown="Disabled" {
          disable-tunnel: [w415 w431] -> w401
          disable-tunnel: [w414 w432] -> w400
          disable-tunnel: w398 -> [w409 w432]
          disable-tunnel: w397 -> [w405 w431]
          frame Disabled {
            n153 = call "Timer2.vi"("error in (no error)"=w405, "Reset"=TRUE) -> ("error out"=w404:errorcluster)  [unwired: 7 in, 2 out]
            n154 = while {
              tunnel: w409 -> [w421]
              tunnel: [w421] -> w408
              tunnel: [w419] -> w407
              tunnel: w404 -> [w420]
              stop <- w418 stop-if-true
              n155 = call "Timer2.vi"("error in (no error)"=w420, "Time Target (s)"=0.25, "Pause"=TRUE) -> ("error out"=w419:errorcluster, "Time has Elapsed"=w418:bool)  [unwired: 6 in, 1 out]
            }
            n156 = property class="Instr"(reference=w408, error in=w407) -> (reference out=w412:refnum<visa-resource-name>, error out=w411:errorcluster, "Bytes at Port"=w410:u32)
            n157 = for {
              N: w410 -> [_]
              tunnel: w411 -> [w429]
              tunnel: w412 -> [w428]
              shift-right: [w423] -> _
              shift-left: "" -> [w427]
              tunnel: [w426] -> w415
              tunnel: [w425] -> w414
              n158 = VISA Read(VISA resource name=w428, byte count=u32 1, error in (no error)=w429) -> (VISA resource name out=w425:refnum<visa-resource-name>, read buffer=w422:string, error out=w426:errorcluster)  [unwired: 1 out]
              n159 = Concatenate Strings(w427, w422) -> (w423:string)
              n160 = Wait Until Next ms Multiple(millisecond multiple=u32 5) -> ()  [unwired: 1 out]
            }
          }
          frame Enabled {
          }
        }
      }
      frame "Gluteos" {
        n161 = Unbundle By Name(w444) -> ("Gluteos"=w442:i32)
        n162 = To Unsigned Byte Integer(number=w442) -> (unsigned 8bit integer=w443:u8)
        n163 = Build Array(w443) -> (w448:u8[])
        n164 = Byte Array To String(unsigned byte array=w448) -> (string=w446:string)
        n165 = Concatenate Strings("3", w446) -> (w445:string)
        n166 = String Length(string=w445) -> (length=w451:i32)
        n167 = for {
          N: w451 -> [_]
          tunnel: w454 -> [w493]
          tunnel: w455 -> [w492]
          tunnel: w445 -> [w489]
          tunnel: [w486] -> w449
          tunnel: [w485] -> w450
          i -> [w487]
          n168 = String Subset(string=w489, offset (0)=w487, length (rest)=1 ("length (rest)")) -> (substring=w490:string)
          n169 = VISA Write(VISA resource name=w492, write buffer=w490, error in (no error)=w493) -> (VISA resource name out=w485:refnum<visa-resource-name>, error out=w486:errorcluster)  [unwired: 1 out]
          n170 = Wait Until Next ms Multiple(millisecond multiple=u32 5) -> ()  [unwired: 1 out]
        }
        n171 = disable-structure shown="Disabled" {
          disable-tunnel: [w467 w483] -> w453
          disable-tunnel: [w466 w484] -> w452
          disable-tunnel: w450 -> [w461 w484]
          disable-tunnel: w449 -> [w457 w483]
          frame Disabled {
            n172 = call "Timer2.vi"("error in (no error)"=w457, "Reset"=TRUE) -> ("error out"=w456:errorcluster)  [unwired: 7 in, 2 out]
            n173 = while {
              tunnel: w461 -> [w473]
              tunnel: [w473] -> w460
              tunnel: [w471] -> w459
              tunnel: w456 -> [w472]
              stop <- w470 stop-if-true
              n174 = call "Timer2.vi"("error in (no error)"=w472, "Time Target (s)"=0.25, "Pause"=TRUE) -> ("error out"=w471:errorcluster, "Time has Elapsed"=w470:bool)  [unwired: 6 in, 1 out]
            }
            n175 = property class="Instr"(reference=w460, error in=w459) -> (reference out=w464:refnum<visa-resource-name>, error out=w463:errorcluster, "Bytes at Port"=w462:u32)
            n176 = for {
              N: w462 -> [_]
              tunnel: w463 -> [w481]
              tunnel: w464 -> [w480]
              shift-right: [w475] -> _
              shift-left: "" -> [w479]
              tunnel: [w478] -> w467
              tunnel: [w477] -> w466
              n177 = VISA Read(VISA resource name=w480, byte count=u32 1, error in (no error)=w481) -> (VISA resource name out=w477:refnum<visa-resource-name>, read buffer=w474:string, error out=w478:errorcluster)  [unwired: 1 out]
              n178 = Concatenate Strings(w479, w474) -> (w475:string)
              n179 = Wait Until Next ms Multiple(millisecond multiple=u32 5) -> ()  [unwired: 1 out]
            }
          }
          frame Enabled {
          }
        }
      }
      frame "Abdomen" {
        n180 = Unbundle By Name(w496) -> ("Abdomen"=w494:i32)
        n181 = To Unsigned Byte Integer(number=w494) -> (unsigned 8bit integer=w495:u8)
        n182 = Build Array(w495) -> (w500:u8[])
        n183 = Byte Array To String(unsigned byte array=w500) -> (string=w498:string)
        n184 = Concatenate Strings("4", w498) -> (w497:string)
        n185 = String Length(string=w497) -> (length=w503:i32)
        n186 = for {
          N: w503 -> [_]
          tunnel: w506 -> [w545]
          tunnel: w507 -> [w544]
          tunnel: w497 -> [w541]
          tunnel: [w538] -> w501
          tunnel: [w537] -> w502
          i -> [w539]
          n187 = String Subset(string=w541, offset (0)=w539, length (rest)=1 ("length (rest)")) -> (substring=w542:string)
          n188 = VISA Write(VISA resource name=w544, write buffer=w542, error in (no error)=w545) -> (VISA resource name out=w537:refnum<visa-resource-name>, error out=w538:errorcluster)  [unwired: 1 out]
          n189 = Wait Until Next ms Multiple(millisecond multiple=u32 5) -> ()  [unwired: 1 out]
        }
        n190 = disable-structure shown="Disabled" {
          disable-tunnel: [w519 w535] -> w505
          disable-tunnel: [w518 w536] -> w504
          disable-tunnel: w502 -> [w513 w536]
          disable-tunnel: w501 -> [w509 w535]
          frame Disabled {
            n191 = call "Timer2.vi"("error in (no error)"=w509, "Reset"=TRUE) -> ("error out"=w508:errorcluster)  [unwired: 7 in, 2 out]
            n192 = while {
              tunnel: w513 -> [w525]
              tunnel: [w525] -> w512
              tunnel: [w523] -> w511
              tunnel: w508 -> [w524]
              stop <- w522 stop-if-true
              n193 = call "Timer2.vi"("error in (no error)"=w524, "Time Target (s)"=0.25, "Pause"=TRUE) -> ("error out"=w523:errorcluster, "Time has Elapsed"=w522:bool)  [unwired: 6 in, 1 out]
            }
            n194 = property class="Instr"(reference=w512, error in=w511) -> (reference out=w516:refnum<visa-resource-name>, error out=w515:errorcluster, "Bytes at Port"=w514:u32)
            n195 = for {
              N: w514 -> [_]
              tunnel: w515 -> [w533]
              tunnel: w516 -> [w532]
              shift-right: [w527] -> _
              shift-left: "" -> [w531]
              tunnel: [w530] -> w519
              tunnel: [w529] -> w518
              n196 = VISA Read(VISA resource name=w532, byte count=u32 1, error in (no error)=w533) -> (VISA resource name out=w529:refnum<visa-resource-name>, read buffer=w526:string, error out=w530:errorcluster)  [unwired: 1 out]
              n197 = Concatenate Strings(w531, w526) -> (w527:string)
              n198 = Wait Until Next ms Multiple(millisecond multiple=u32 5) -> ()  [unwired: 1 out]
            }
          }
          frame Enabled {
          }
        }
      }
      frame "Lumbares" {
        n199 = Unbundle By Name(w548) -> ("Lumbares"=w546:i32)
        n200 = To Unsigned Byte Integer(number=w546) -> (unsigned 8bit integer=w547:u8)
        n201 = Build Array(w547) -> (w552:u8[])
        n202 = Byte Array To String(unsigned byte array=w552) -> (string=w550:string)
        n203 = Concatenate Strings("5", w550) -> (w549:string)
        n204 = String Length(string=w549) -> (length=w555:i32)
        n205 = for {
          N: w555 -> [_]
          tunnel: w558 -> [w597]
          tunnel: w559 -> [w596]
          tunnel: w549 -> [w593]
          tunnel: [w590] -> w553
          tunnel: [w589] -> w554
          i -> [w591]
          n206 = String Subset(string=w593, offset (0)=w591, length (rest)=1 ("length (rest)")) -> (substring=w594:string)
          n207 = VISA Write(VISA resource name=w596, write buffer=w594, error in (no error)=w597) -> (VISA resource name out=w589:refnum<visa-resource-name>, error out=w590:errorcluster)  [unwired: 1 out]
          n208 = Wait Until Next ms Multiple(millisecond multiple=u32 5) -> ()  [unwired: 1 out]
        }
        n209 = disable-structure shown="Disabled" {
          disable-tunnel: [w571 w587] -> w557
          disable-tunnel: [w570 w588] -> w556
          disable-tunnel: w554 -> [w565 w588]
          disable-tunnel: w553 -> [w561 w587]
          frame Disabled {
            n210 = call "Timer2.vi"("error in (no error)"=w561, "Reset"=TRUE) -> ("error out"=w560:errorcluster)  [unwired: 7 in, 2 out]
            n211 = while {
              tunnel: w565 -> [w577]
              tunnel: [w577] -> w564
              tunnel: [w575] -> w563
              tunnel: w560 -> [w576]
              stop <- w574 stop-if-true
              n212 = call "Timer2.vi"("error in (no error)"=w576, "Time Target (s)"=0.25, "Pause"=TRUE) -> ("error out"=w575:errorcluster, "Time has Elapsed"=w574:bool)  [unwired: 6 in, 1 out]
            }
            n213 = property class="Instr"(reference=w564, error in=w563) -> (reference out=w568:refnum<visa-resource-name>, error out=w567:errorcluster, "Bytes at Port"=w566:u32)
            n214 = for {
              N: w566 -> [_]
              tunnel: w567 -> [w585]
              tunnel: w568 -> [w584]
              shift-right: [w579] -> _
              shift-left: "" -> [w583]
              tunnel: [w582] -> w571
              tunnel: [w581] -> w570
              n215 = VISA Read(VISA resource name=w584, byte count=u32 1, error in (no error)=w585) -> (VISA resource name out=w581:refnum<visa-resource-name>, read buffer=w578:string, error out=w582:errorcluster)  [unwired: 1 out]
              n216 = Concatenate Strings(w583, w578) -> (w579:string)
              n217 = Wait Until Next ms Multiple(millisecond multiple=u32 5) -> ()  [unwired: 1 out]
            }
          }
          frame Enabled {
          }
        }
      }
      frame "Dorsales" {
        n218 = Unbundle By Name(w600) -> ("Dorsales"=w598:i32)
        n219 = To Unsigned Byte Integer(number=w598) -> (unsigned 8bit integer=w599:u8)
        n220 = Build Array(w599) -> (w604:u8[])
        n221 = Byte Array To String(unsigned byte array=w604) -> (string=w602:string)
        n222 = Concatenate Strings("6", w602) -> (w601:string)
        n223 = String Length(string=w601) -> (length=w607:i32)
        n224 = for {
          N: w607 -> [_]
          tunnel: w610 -> [w649]
          tunnel: w611 -> [w648]
          tunnel: w601 -> [w645]
          tunnel: [w642] -> w605
          tunnel: [w641] -> w606
          i -> [w643]
          n225 = String Subset(string=w645, offset (0)=w643, length (rest)=1 ("length (rest)")) -> (substring=w646:string)
          n226 = VISA Write(VISA resource name=w648, write buffer=w646, error in (no error)=w649) -> (VISA resource name out=w641:refnum<visa-resource-name>, error out=w642:errorcluster)  [unwired: 1 out]
          n227 = Wait Until Next ms Multiple(millisecond multiple=u32 5) -> ()  [unwired: 1 out]
        }
        n228 = disable-structure shown="Disabled" {
          disable-tunnel: [w623 w639] -> w609
          disable-tunnel: [w622 w640] -> w608
          disable-tunnel: w606 -> [w617 w640]
          disable-tunnel: w605 -> [w613 w639]
          frame Disabled {
            n229 = call "Timer2.vi"("error in (no error)"=w613, "Reset"=TRUE) -> ("error out"=w612:errorcluster)  [unwired: 7 in, 2 out]
            n230 = while {
              tunnel: w617 -> [w629]
              tunnel: [w629] -> w616
              tunnel: [w627] -> w615
              tunnel: w612 -> [w628]
              stop <- w626 stop-if-true
              n231 = call "Timer2.vi"("error in (no error)"=w628, "Time Target (s)"=0.25, "Pause"=TRUE) -> ("error out"=w627:errorcluster, "Time has Elapsed"=w626:bool)  [unwired: 6 in, 1 out]
            }
            n232 = property class="Instr"(reference=w616, error in=w615) -> (reference out=w620:refnum<visa-resource-name>, error out=w619:errorcluster, "Bytes at Port"=w618:u32)
            n233 = for {
              N: w618 -> [_]
              tunnel: w619 -> [w637]
              tunnel: w620 -> [w636]
              shift-right: [w631] -> _
              shift-left: "" -> [w635]
              tunnel: [w634] -> w623
              tunnel: [w633] -> w622
              n234 = VISA Read(VISA resource name=w636, byte count=u32 1, error in (no error)=w637) -> (VISA resource name out=w633:refnum<visa-resource-name>, read buffer=w630:string, error out=w634:errorcluster)  [unwired: 1 out]
              n235 = Concatenate Strings(w635, w630) -> (w631:string)
              n236 = Wait Until Next ms Multiple(millisecond multiple=u32 5) -> ()  [unwired: 1 out]
            }
          }
          frame Enabled {
          }
        }
      }
      frame "Trapecio" {
        n237 = Unbundle By Name(w652) -> ("Trapecio"=w650:i32)
        n238 = To Unsigned Byte Integer(number=w650) -> (unsigned 8bit integer=w651:u8)
        n239 = Build Array(w651) -> (w656:u8[])
        n240 = Byte Array To String(unsigned byte array=w656) -> (string=w654:string)
        n241 = Concatenate Strings("7", w654) -> (w653:string)
        n242 = String Length(string=w653) -> (length=w659:i32)
        n243 = for {
          N: w659 -> [_]
          tunnel: w662 -> [w701]
          tunnel: w663 -> [w700]
          tunnel: w653 -> [w697]
          tunnel: [w694] -> w657
          tunnel: [w693] -> w658
          i -> [w695]
          n244 = String Subset(string=w697, offset (0)=w695, length (rest)=1 ("length (rest)")) -> (substring=w698:string)
          n245 = VISA Write(VISA resource name=w700, write buffer=w698, error in (no error)=w701) -> (VISA resource name out=w693:refnum<visa-resource-name>, error out=w694:errorcluster)  [unwired: 1 out]
          n246 = Wait Until Next ms Multiple(millisecond multiple=u32 5) -> ()  [unwired: 1 out]
        }
        n247 = disable-structure shown="Disabled" {
          disable-tunnel: [w675 w691] -> w661
          disable-tunnel: [w674 w692] -> w660
          disable-tunnel: w658 -> [w669 w692]
          disable-tunnel: w657 -> [w665 w691]
          frame Disabled {
            n248 = call "Timer2.vi"("error in (no error)"=w665, "Reset"=TRUE) -> ("error out"=w664:errorcluster)  [unwired: 7 in, 2 out]
            n249 = while {
              tunnel: w669 -> [w681]
              tunnel: [w681] -> w668
              tunnel: [w679] -> w667
              tunnel: w664 -> [w680]
              stop <- w678 stop-if-true
              n250 = call "Timer2.vi"("error in (no error)"=w680, "Time Target (s)"=0.25, "Pause"=TRUE) -> ("error out"=w679:errorcluster, "Time has Elapsed"=w678:bool)  [unwired: 6 in, 1 out]
            }
            n251 = property class="Instr"(reference=w668, error in=w667) -> (reference out=w672:refnum<visa-resource-name>, error out=w671:errorcluster, "Bytes at Port"=w670:u32)
            n252 = for {
              N: w670 -> [_]
              tunnel: w671 -> [w689]
              tunnel: w672 -> [w688]
              shift-right: [w683] -> _
              shift-left: "" -> [w687]
              tunnel: [w686] -> w675
              tunnel: [w685] -> w674
              n253 = VISA Read(VISA resource name=w688, byte count=u32 1, error in (no error)=w689) -> (VISA resource name out=w685:refnum<visa-resource-name>, read buffer=w682:string, error out=w686:errorcluster)  [unwired: 1 out]
              n254 = Concatenate Strings(w687, w682) -> (w683:string)
              n255 = Wait Until Next ms Multiple(millisecond multiple=u32 5) -> ()  [unwired: 1 out]
            }
          }
          frame Enabled {
          }
        }
      }
      frame "Pectorales" {
        n256 = Unbundle By Name(w704) -> ("Pectorales"=w702:i32)
        n257 = To Unsigned Byte Integer(number=w702) -> (unsigned 8bit integer=w703:u8)
        n258 = Build Array(w703) -> (w708:u8[])
        n259 = Byte Array To String(unsigned byte array=w708) -> (string=w706:string)
        n260 = Concatenate Strings("8", w706) -> (w705:string)
        n261 = String Length(string=w705) -> (length=w711:i32)
        n262 = for {
          N: w711 -> [_]
          tunnel: w714 -> [w753]
          tunnel: w715 -> [w752]
          tunnel: w705 -> [w749]
          tunnel: [w746] -> w709
          tunnel: [w745] -> w710
          i -> [w747]
          n263 = String Subset(string=w749, offset (0)=w747, length (rest)=1 ("length (rest)")) -> (substring=w750:string)
          n264 = VISA Write(VISA resource name=w752, write buffer=w750, error in (no error)=w753) -> (VISA resource name out=w745:refnum<visa-resource-name>, error out=w746:errorcluster)  [unwired: 1 out]
          n265 = Wait Until Next ms Multiple(millisecond multiple=u32 5) -> ()  [unwired: 1 out]
        }
        n266 = disable-structure shown="Disabled" {
          disable-tunnel: [w727 w743] -> w713
          disable-tunnel: [w726 w744] -> w712
          disable-tunnel: w710 -> [w721 w744]
          disable-tunnel: w709 -> [w717 w743]
          frame Disabled {
            n267 = call "Timer2.vi"("error in (no error)"=w717, "Reset"=TRUE) -> ("error out"=w716:errorcluster)  [unwired: 7 in, 2 out]
            n268 = while {
              tunnel: w721 -> [w733]
              tunnel: [w733] -> w720
              tunnel: [w731] -> w719
              tunnel: w716 -> [w732]
              stop <- w730 stop-if-true
              n269 = call "Timer2.vi"("error in (no error)"=w732, "Time Target (s)"=0.25, "Pause"=TRUE) -> ("error out"=w731:errorcluster, "Time has Elapsed"=w730:bool)  [unwired: 6 in, 1 out]
            }
            n270 = property class="Instr"(reference=w720, error in=w719) -> (reference out=w724:refnum<visa-resource-name>, error out=w723:errorcluster, "Bytes at Port"=w722:u32)
            n271 = for {
              N: w722 -> [_]
              tunnel: w723 -> [w741]
              tunnel: w724 -> [w740]
              shift-right: [w735] -> _
              shift-left: "" -> [w739]
              tunnel: [w738] -> w727
              tunnel: [w737] -> w726
              n272 = VISA Read(VISA resource name=w740, byte count=u32 1, error in (no error)=w741) -> (VISA resource name out=w737:refnum<visa-resource-name>, read buffer=w734:string, error out=w738:errorcluster)  [unwired: 1 out]
              n273 = Concatenate Strings(w739, w734) -> (w735:string)
              n274 = Wait Until Next ms Multiple(millisecond multiple=u32 5) -> ()  [unwired: 1 out]
            }
          }
          frame Enabled {
          }
        }
      }
      frame "Biceps" {
        n275 = Unbundle By Name(w756) -> ("Biceps"=w754:i32)
        n276 = To Unsigned Byte Integer(number=w754) -> (unsigned 8bit integer=w755:u8)
        n277 = Build Array(w755) -> (w760:u8[])
        n278 = Byte Array To String(unsigned byte array=w760) -> (string=w758:string)
        n279 = Concatenate Strings("9", w758) -> (w757:string)
        n280 = String Length(string=w757) -> (length=w763:i32)
        n281 = for {
          N: w763 -> [_]
          tunnel: w766 -> [w805]
          tunnel: w767 -> [w804]
          tunnel: w757 -> [w801]
          tunnel: [w798] -> w761
          tunnel: [w797] -> w762
          i -> [w799]
          n282 = String Subset(string=w801, offset (0)=w799, length (rest)=1 ("length (rest)")) -> (substring=w802:string)
          n283 = VISA Write(VISA resource name=w804, write buffer=w802, error in (no error)=w805) -> (VISA resource name out=w797:refnum<visa-resource-name>, error out=w798:errorcluster)  [unwired: 1 out]
          n284 = Wait Until Next ms Multiple(millisecond multiple=u32 5) -> ()  [unwired: 1 out]
        }
        n285 = disable-structure shown="Disabled" {
          disable-tunnel: [w779 w795] -> w765
          disable-tunnel: [w778 w796] -> w764
          disable-tunnel: w762 -> [w773 w796]
          disable-tunnel: w761 -> [w769 w795]
          frame Disabled {
            n286 = call "Timer2.vi"("error in (no error)"=w769, "Reset"=TRUE) -> ("error out"=w768:errorcluster)  [unwired: 7 in, 2 out]
            n287 = while {
              tunnel: w773 -> [w785]
              tunnel: [w785] -> w772
              tunnel: [w783] -> w771
              tunnel: w768 -> [w784]
              stop <- w782 stop-if-true
              n288 = call "Timer2.vi"("error in (no error)"=w784, "Time Target (s)"=0.25, "Pause"=TRUE) -> ("error out"=w783:errorcluster, "Time has Elapsed"=w782:bool)  [unwired: 6 in, 1 out]
            }
            n289 = property class="Instr"(reference=w772, error in=w771) -> (reference out=w776:refnum<visa-resource-name>, error out=w775:errorcluster, "Bytes at Port"=w774:u32)
            n290 = for {
              N: w774 -> [_]
              tunnel: w775 -> [w793]
              tunnel: w776 -> [w792]
              shift-right: [w787] -> _
              shift-left: "" -> [w791]
              tunnel: [w790] -> w779
              tunnel: [w789] -> w778
              n291 = VISA Read(VISA resource name=w792, byte count=u32 1, error in (no error)=w793) -> (VISA resource name out=w789:refnum<visa-resource-name>, read buffer=w786:string, error out=w790:errorcluster)  [unwired: 1 out]
              n292 = Concatenate Strings(w791, w786) -> (w787:string)
              n293 = Wait Until Next ms Multiple(millisecond multiple=u32 5) -> ()  [unwired: 1 out]
            }
          }
          frame Enabled {
          }
        }
      }
      frame "Opcional" {
        n294 = Unbundle By Name(w808) -> ("Opcional"=w806:i32)
        n295 = To Unsigned Byte Integer(number=w806) -> (unsigned 8bit integer=w807:u8)
        n296 = Build Array(w807) -> (w812:u8[])
        n297 = Byte Array To String(unsigned byte array=w812) -> (string=w810:string)
        n298 = Concatenate Strings("10", w810) -> (w809:string)
        n299 = String Length(string=w809) -> (length=w815:i32)
        n300 = for {
          N: w815 -> [_]
          tunnel: w818 -> [w857]
          tunnel: w819 -> [w856]
          tunnel: w809 -> [w853]
          tunnel: [w850] -> w813
          tunnel: [w849] -> w814
          i -> [w851]
          n301 = String Subset(string=w853, offset (0)=w851, length (rest)=1 ("length (rest)")) -> (substring=w854:string)
          n302 = VISA Write(VISA resource name=w856, write buffer=w854, error in (no error)=w857) -> (VISA resource name out=w849:refnum<visa-resource-name>, error out=w850:errorcluster)  [unwired: 1 out]
          n303 = Wait Until Next ms Multiple(millisecond multiple=u32 5) -> ()  [unwired: 1 out]
        }
        n304 = disable-structure shown="Disabled" {
          disable-tunnel: [w831 w847] -> w817
          disable-tunnel: [w830 w848] -> w816
          disable-tunnel: w814 -> [w825 w848]
          disable-tunnel: w813 -> [w821 w847]
          frame Disabled {
            n305 = call "Timer2.vi"("error in (no error)"=w821, "Reset"=TRUE) -> ("error out"=w820:errorcluster)  [unwired: 7 in, 2 out]
            n306 = while {
              tunnel: w825 -> [w837]
              tunnel: [w837] -> w824
              tunnel: [w835] -> w823
              tunnel: w820 -> [w836]
              stop <- w834 stop-if-true
              n307 = call "Timer2.vi"("error in (no error)"=w836, "Time Target (s)"=0.25, "Pause"=TRUE) -> ("error out"=w835:errorcluster, "Time has Elapsed"=w834:bool)  [unwired: 6 in, 1 out]
            }
            n308 = property class="Instr"(reference=w824, error in=w823) -> (reference out=w828:refnum<visa-resource-name>, error out=w827:errorcluster, "Bytes at Port"=w826:u32)
            n309 = for {
              N: w826 -> [_]
              tunnel: w827 -> [w845]
              tunnel: w828 -> [w844]
              shift-right: [w839] -> _
              shift-left: "" -> [w843]
              tunnel: [w842] -> w831
              tunnel: [w841] -> w830
              n310 = VISA Read(VISA resource name=w844, byte count=u32 1, error in (no error)=w845) -> (VISA resource name out=w841:refnum<visa-resource-name>, read buffer=w838:string, error out=w842:errorcluster)  [unwired: 1 out]
              n311 = Concatenate Strings(w843, w838) -> (w839:string)
              n312 = Wait Until Next ms Multiple(millisecond multiple=u32 5) -> ()  [unwired: 1 out]
            }
          }
          frame Enabled {
          }
        }
      }
    }
    n313 = local read "Stop"() -> (w66:bool)
    n314 = local read "Back"() -> (w67:bool)
    n315 = Or(x=w66, y=w67) -> (x .or. y?=w65:bool)
  }
  n316 = while {
    tunnel: w2 -> [w861]
    shift-right: [w859] -> _
    shift-left: w3 -> [w860]
    tunnel: w7 -> [w858]
    stop <- w862 stop-if-true
    n317 = event shown="[0] \"Cuadriceps Bool\": Value Change" {
      selector: _ -> [_ _ _ _ _ _ _ _ _ _ _ _ _ _ _ _ _ _ _ _]
      dyn-events: _ -> [_ _ _ _ _ _ _ _ _ _ _ _ _ _ _ _ _ _ _ _]
      timeout: _ -> [_ _ _ _ _ _ _ _ _ _ _ _ _ _ _ _ _ _ _ _]
      tunnel: [FALSE FALSE FALSE FALSE FALSE FALSE FALSE FALSE FALSE FALSE _ _ _ "Stop" TRUE ("Stop") FALSE ("Stop") FALSE ("Stop") FALSE ("Stop") FALSE ("Stop") FALSE ("Stop")] -> w862
      tunnel: w861 -> [_ _ _ _ _ _ _ _ _ _ w1003 w1153 w1268 _ _ _ _ w1387 w1440 _]
      tunnel: w860 -> [w863 w877 w892 w906 w920 w934 w948 w962 w976 w990 w1006 w1155 w1272 w1341 w1345 w1356 w1372 w1389 w1441 w1446]
      tunnel: [w864 w878 w891 w905 w919 w933 w947 w961 w975 w989 w1007 w1156 w1273 w1341 w1343 w1354 w1372 w1375 w1392 w1445] -> w859
      tunnel: w858 -> [_ _ _ _ _ _ _ _ _ _ w1004 w1152 w1269 _ _ _ _ w1386 w1439 _]
      event "Cuadriceps Bool": Value Change {
        n318 = event-data() -> ()  [unwired: 1 in, 6 out]
        n319 = Bundle By Name(cluster=cluster{"Color Box":u32, "Color Box 2":u32} {"Color Box"=12369084, "Color Box 2"=12369084}, "Color Box"=u32 16711680 ("Color Box 2")) -> (w873:cluster{"Color Box":u32, "Color Box 2":u32})
        n320 = Bundle By Name(cluster=cluster{"Color Box":u32, "Color Box 2":u32} {"Color Box"=12369084, "Color Box 2"=12369084}, "Color Box"=u32 12369084 ("Color Box 2")) -> (w868:cluster{"Color Box":u32, "Color Box 2":u32})
        n321 = Bundle By Name(cluster=w863, "Label"="Cuadriceps" ("Message")) -> (w864:T1)
        n322 = Insert Into Array(array=cluster{u32, u32}[] [] ("Colors [4]"), new element=w873) -> (w872:cluster{u32, u32}[])  [unwired: 1 in]
        n323 = Insert Into Array(array=cluster{u32, u32}[] [] ("Colors [4]"), new element=w868) -> (w866:cluster{u32, u32}[])  [unwired: 1 in]
        n324 = property on="Cuadriceps Bool" class="Bool"("Colors [4]"=w872) -> ()  [unwired: 2 in, 2 out]
        n325 = property on="Abdomen Bool" class="Bool"("Colors [4]"=w866) -> ()  [unwired: 2 in, 2 out]
        n326 = property on="Lumbares Bool" class="Bool"("Colors [4]"=w866) -> ()  [unwired: 2 in, 2 out]
        n327 = property on="Gluteos Bool" class="Bool"("Colors [4]"=w866) -> ()  [unwired: 2 in, 2 out]
        n328 = property on="Isquiotibiales Bool" class="Bool"("Colors [4]"=w866) -> ()  [unwired: 2 in, 2 out]
        n329 = property on="Pectorales Bool" class="Bool"("Colors [4]"=w866) -> ()  [unwired: 2 in, 2 out]
        n330 = property on="Dorsales Bool" class="Bool"("Colors [4]"=w866) -> ()  [unwired: 2 in, 2 out]
        n331 = property on="Trapecio Bool" class="Bool"("Colors [4]"=w866) -> ()  [unwired: 2 in, 2 out]
        n332 = property on="Opcional Bool" class="Bool"("Colors [4]"=w866) -> ()  [unwired: 2 in, 2 out]
        n333 = property on="Biceps Bool" class="Bool"("Colors [4]"=w866) -> ()  [unwired: 2 in, 2 out]
      }
      event "Isquiotibiales Bool": Value Change {
        n334 = event-data() -> ()  [unwired: 1 in, 6 out]
        n335 = Bundle By Name(cluster=cluster{"Color Box":u32, "Color Box 2":u32} {"Color Box"=12369084, "Color Box 2"=12369084}, "Color Box"=u32 16711680 ("Color Box 2")) -> (w887:cluster{"Color Box":u32, "Color Box 2":u32})
        n336 = Bundle By Name(cluster=cluster{"Color Box":u32, "Color Box 2":u32} {"Color Box"=12369084, "Color Box 2"=12369084}, "Color Box"=u32 12369084 ("Color Box 2")) -> (w883:cluster{"Color Box":u32, "Color Box 2":u32})
        n337 = Bundle By Name(cluster=w877, "Label"="Isquiotibiales" ("Message")) -> (w878:T1)
        n338 = Insert Into Array(array=cluster{u32, u32}[] [] ("Colors [4]"), new element=w887) -> (w881:cluster{u32, u32}[])  [unwired: 1 in]
        n339 = Insert Into Array(array=cluster{u32, u32}[] [] ("Colors [4]"), new element=w883) -> (w880:cluster{u32, u32}[])  [unwired: 1 in]
        n340 = property on="Isquiotibiales Bool" class="Bool"("Colors [4]"=w881) -> ()  [unwired: 2 in, 2 out]
        n341 = property on="Abdomen Bool" class="Bool"("Colors [4]"=w880) -> ()  [unwired: 2 in, 2 out]
        n342 = property on="Lumbares Bool" class="Bool"("Colors [4]"=w880) -> ()  [unwired: 2 in, 2 out]
        n343 = property on="Gluteos Bool" class="Bool"("Colors [4]"=w880) -> ()  [unwired: 2 in, 2 out]
        n344 = property on="Cuadriceps Bool" class="Bool"("Colors [4]"=w880) -> ()  [unwired: 2 in, 2 out]
        n345 = property on="Pectorales Bool" class="Bool"("Colors [4]"=w880) -> ()  [unwired: 2 in, 2 out]
        n346 = property on="Dorsales Bool" class="Bool"("Colors [4]"=w880) -> ()  [unwired: 2 in, 2 out]
        n347 = property on="Trapecio Bool" class="Bool"("Colors [4]"=w880) -> ()  [unwired: 2 in, 2 out]
        n348 = property on="Opcional Bool" class="Bool"("Colors [4]"=w880) -> ()  [unwired: 2 in, 2 out]
        n349 = property on="Biceps Bool" class="Bool"("Colors [4]"=w880) -> ()  [unwired: 2 in, 2 out]
      }
      event "Gluteos Bool": Value Change {
        n350 = event-data() -> ()  [unwired: 1 in, 6 out]
        n351 = Bundle By Name(cluster=cluster{"Color Box":u32, "Color Box 2":u32} {"Color Box"=12369084, "Color Box 2"=12369084}, "Color Box"=u32 16711680 ("Color Box 2")) -> (w901:cluster{"Color Box":u32, "Color Box 2":u32})
        n352 = Bundle By Name(cluster=cluster{"Color Box":u32, "Color Box 2":u32} {"Color Box"=12369084, "Color Box 2"=12369084}, "Color Box"=u32 12369084 ("Color Box 2")) -> (w897:cluster{"Color Box":u32, "Color Box 2":u32})
        n353 = Bundle By Name(cluster=w892, "Label"="Gluteos" ("Message")) -> (w891:T1)
        n354 = Insert Into Array(array=cluster{u32, u32}[] [] ("Colors [4]"), new element=w901) -> (w895:cluster{u32, u32}[])  [unwired: 1 in]
        n355 = Insert Into Array(array=cluster{u32, u32}[] [] ("Colors [4]"), new element=w897) -> (w894:cluster{u32, u32}[])  [unwired: 1 in]
        n356 = property on="Gluteos Bool" class="Bool"("Colors [4]"=w895) -> ()  [unwired: 2 in, 2 out]
        n357 = property on="Abdomen Bool" class="Bool"("Colors [4]"=w894) -> ()  [unwired: 2 in, 2 out]
        n358 = property on="Lumbares Bool" class="Bool"("Colors [4]"=w894) -> ()  [unwired: 2 in, 2 out]
        n359 = property on="Isquiotibiales Bool" class="Bool"("Colors [4]"=w894) -> ()  [unwired: 2 in, 2 out]
        n360 = property on="Cuadriceps Bool" class="Bool"("Colors [4]"=w894) -> ()  [unwired: 2 in, 2 out]
        n361 = property on="Pectorales Bool" class="Bool"("Colors [4]"=w894) -> ()  [unwired: 2 in, 2 out]
        n362 = property on="Dorsales Bool" class="Bool"("Colors [4]"=w894) -> ()  [unwired: 2 in, 2 out]
        n363 = property on="Trapecio Bool" class="Bool"("Colors [4]"=w894) -> ()  [unwired: 2 in, 2 out]
        n364 = property on="Opcional Bool" class="Bool"("Colors [4]"=w894) -> ()  [unwired: 2 in, 2 out]
        n365 = property on="Biceps Bool" class="Bool"("Colors [4]"=w894) -> ()  [unwired: 2 in, 2 out]
      }
      event "Abdomen Bool": Value Change {
        n366 = event-data() -> ()  [unwired: 1 in, 6 out]
        n367 = Bundle By Name(cluster=cluster{"Color Box":u32, "Color Box 2":u32} {"Color Box"=12369084, "Color Box 2"=12369084}, "Color Box"=u32 16711680 ("Color Box 2")) -> (w915:cluster{"Color Box":u32, "Color Box 2":u32})
        n368 = Bundle By Name(cluster=cluster{"Color Box":u32, "Color Box 2":u32} {"Color Box"=12369084, "Color Box 2"=12369084}, "Color Box"=u32 12369084 ("Color Box 2")) -> (w911:cluster{"Color Box":u32, "Color Box 2":u32})
        n369 = Bundle By Name(cluster=w906, "Label"="Abdomen" ("Message")) -> (w905:T1)
        n370 = Insert Into Array(array=cluster{u32, u32}[] [] ("Colors [4]"), new element=w915) -> (w909:cluster{u32, u32}[])  [unwired: 1 in]
        n371 = Insert Into Array(array=cluster{u32, u32}[] [] ("Colors [4]"), new element=w911) -> (w908:cluster{u32, u32}[])  [unwired: 1 in]
        n372 = property on="Abdomen Bool" class="Bool"("Colors [4]"=w909) -> ()  [unwired: 2 in, 2 out]
        n373 = property on="Gluteos Bool" class="Bool"("Colors [4]"=w908) -> ()  [unwired: 2 in, 2 out]
        n374 = property on="Lumbares Bool" class="Bool"("Colors [4]"=w908) -> ()  [unwired: 2 in, 2 out]
        n375 = property on="Isquiotibiales Bool" class="Bool"("Colors [4]"=w908) -> ()  [unwired: 2 in, 2 out]
        n376 = property on="Cuadriceps Bool" class="Bool"("Colors [4]"=w908) -> ()  [unwired: 2 in, 2 out]
        n377 = property on="Pectorales Bool" class="Bool"("Colors [4]"=w908) -> ()  [unwired: 2 in, 2 out]
        n378 = property on="Dorsales Bool" class="Bool"("Colors [4]"=w908) -> ()  [unwired: 2 in, 2 out]
        n379 = property on="Trapecio Bool" class="Bool"("Colors [4]"=w908) -> ()  [unwired: 2 in, 2 out]
        n380 = property on="Opcional Bool" class="Bool"("Colors [4]"=w908) -> ()  [unwired: 2 in, 2 out]
        n381 = property on="Biceps Bool" class="Bool"("Colors [4]"=w908) -> ()  [unwired: 2 in, 2 out]
      }
      event "Lumbares Bool": Value Change {
        n382 = event-data() -> ()  [unwired: 1 in, 6 out]
        n383 = Bundle By Name(cluster=cluster{"Color Box":u32, "Color Box 2":u32} {"Color Box"=12369084, "Color Box 2"=12369084}, "Color Box"=u32 16711680 ("Color Box 2")) -> (w929:cluster{"Color Box":u32, "Color Box 2":u32})
        n384 = Bundle By Name(cluster=cluster{"Color Box":u32, "Color Box 2":u32} {"Color Box"=12369084, "Color Box 2"=12369084}, "Color Box"=u32 12369084 ("Color Box 2")) -> (w925:cluster{"Color Box":u32, "Color Box 2":u32})
        n385 = Insert Into Array(array=cluster{u32, u32}[] [] ("Colors [4]"), new element=w929) -> (w923:cluster{u32, u32}[])  [unwired: 1 in]
        n386 = Insert Into Array(array=cluster{u32, u32}[] [] ("Colors [4]"), new element=w925) -> (w922:cluster{u32, u32}[])  [unwired: 1 in]
        n387 = Bundle By Name(cluster=w920, "Label"="Lumbares" ("Message")) -> (w919:T1)
        n388 = property on="Lumbares Bool" class="Bool"("Colors [4]"=w923) -> ()  [unwired: 2 in, 2 out]
        n389 = property on="Gluteos Bool" class="Bool"("Colors [4]"=w922) -> ()  [unwired: 2 in, 2 out]
        n390 = property on="Abdomen Bool" class="Bool"("Colors [4]"=w922) -> ()  [unwired: 2 in, 2 out]
        n391 = property on="Isquiotibiales Bool" class="Bool"("Colors [4]"=w922) -> ()  [unwired: 2 in, 2 out]
        n392 = property on="Cuadriceps Bool" class="Bool"("Colors [4]"=w922) -> ()  [unwired: 2 in, 2 out]
        n393 = property on="Pectorales Bool" class="Bool"("Colors [4]"=w922) -> ()  [unwired: 2 in, 2 out]
        n394 = property on="Dorsales Bool" class="Bool"("Colors [4]"=w922) -> ()  [unwired: 2 in, 2 out]
        n395 = property on="Trapecio Bool" class="Bool"("Colors [4]"=w922) -> ()  [unwired: 2 in, 2 out]
        n396 = property on="Opcional Bool" class="Bool"("Colors [4]"=w922) -> ()  [unwired: 2 in, 2 out]
        n397 = property on="Biceps Bool" class="Bool"("Colors [4]"=w922) -> ()  [unwired: 2 in, 2 out]
      }
      event "Dorsales Bool": Value Change {
        n398 = event-data() -> ()  [unwired: 1 in, 6 out]
        n399 = Bundle By Name(cluster=cluster{"Color Box":u32, "Color Box 2":u32} {"Color Box"=12369084, "Color Box 2"=12369084}, "Color Box"=u32 16711680 ("Color Box 2")) -> (w943:cluster{"Color Box":u32, "Color Box 2":u32})
        n400 = Bundle By Name(cluster=cluster{"Color Box":u32, "Color Box 2":u32} {"Color Box"=12369084, "Color Box 2"=12369084}, "Color Box"=u32 12369084 ("Color Box 2")) -> (w939:cluster{"Color Box":u32, "Color Box 2":u32})
        n401 = Bundle By Name(cluster=w934, "Label"="Dorsales" ("Message")) -> (w933:T1)
        n402 = Insert Into Array(array=cluster{u32, u32}[] [] ("Colors [4]"), new element=w943) -> (w936:cluster{u32, u32}[])  [unwired: 1 in]
        n403 = Insert Into Array(array=cluster{u32, u32}[] [] ("Colors [4]"), new element=w939) -> (w937:cluster{u32, u32}[])  [unwired: 1 in]
        n404 = property on="Gluteos Bool" class="Bool"("Colors [4]"=w937) -> ()  [unwired: 2 in, 2 out]
        n405 = property on="Abdomen Bool" class="Bool"("Colors [4]"=w937) -> ()  [unwired: 2 in, 2 out]
        n406 = property on="Isquiotibiales Bool" class="Bool"("Colors [4]"=w937) -> ()  [unwired: 2 in, 2 out]
        n407 = property on="Cuadriceps Bool" class="Bool"("Colors [4]"=w937) -> ()  [unwired: 2 in, 2 out]
        n408 = property on="Dorsales Bool" class="Bool"("Colors [4]"=w936) -> ()  [unwired: 2 in, 2 out]
        n409 = property on="Pectorales Bool" class="Bool"("Colors [4]"=w937) -> ()  [unwired: 2 in, 2 out]
        n410 = property on="Lumbares Bool" class="Bool"("Colors [4]"=w937) -> ()  [unwired: 2 in, 2 out]
        n411 = property on="Trapecio Bool" class="Bool"("Colors [4]"=w937) -> ()  [unwired: 2 in, 2 out]
        n412 = property on="Opcional Bool" class="Bool"("Colors [4]"=w937) -> ()  [unwired: 2 in, 2 out]
        n413 = property on="Biceps Bool" class="Bool"("Colors [4]"=w937) -> ()  [unwired: 2 in, 2 out]
      }
      event "Trapecio Bool": Value Change {
        n414 = event-data() -> ()  [unwired: 1 in, 6 out]
        n415 = Bundle By Name(cluster=cluster{"Color Box":u32, "Color Box 2":u32} {"Color Box"=12369084, "Color Box 2"=12369084}, "Color Box"=u32 16711680 ("Color Box 2")) -> (w957:cluster{"Color Box":u32, "Color Box 2":u32})
        n416 = Bundle By Name(cluster=cluster{"Color Box":u32, "Color Box 2":u32} {"Color Box"=12369084, "Color Box 2"=12369084}, "Color Box"=u32 12369084 ("Color Box 2")) -> (w953:cluster{"Color Box":u32, "Color Box 2":u32})
        n417 = Bundle By Name(cluster=w948, "Label"="Trapecio" ("Message")) -> (w947:T1)
        n418 = Insert Into Array(array=cluster{u32, u32}[] [] ("Colors [4]"), new element=w957) -> (w950:cluster{u32, u32}[])  [unwired: 1 in]
        n419 = Insert Into Array(array=cluster{u32, u32}[] [] ("Colors [4]"), new element=w953) -> (w951:cluster{u32, u32}[])  [unwired: 1 in]
        n420 = property on="Trapecio Bool" class="Bool"("Colors [4]"=w950) -> ()  [unwired: 2 in, 2 out]
        n421 = property on="Gluteos Bool" class="Bool"("Colors [4]"=w951) -> ()  [unwired: 2 in, 2 out]
        n422 = property on="Abdomen Bool" class="Bool"("Colors [4]"=w951) -> ()  [unwired: 2 in, 2 out]
        n423 = property on="Isquiotibiales Bool" class="Bool"("Colors [4]"=w951) -> ()  [unwired: 2 in, 2 out]
        n424 = property on="Cuadriceps Bool" class="Bool"("Colors [4]"=w951) -> ()  [unwired: 2 in, 2 out]
        n425 = property on="Pectorales Bool" class="Bool"("Colors [4]"=w951) -> ()  [unwired: 2 in, 2 out]
        n426 = property on="Lumbares Bool" class="Bool"("Colors [4]"=w951) -> ()  [unwired: 2 in, 2 out]
        n427 = property on="Dorsales Bool" class="Bool"("Colors [4]"=w951) -> ()  [unwired: 2 in, 2 out]
        n428 = property on="Opcional Bool" class="Bool"("Colors [4]"=w951) -> ()  [unwired: 2 in, 2 out]
        n429 = property on="Biceps Bool" class="Bool"("Colors [4]"=w951) -> ()  [unwired: 2 in, 2 out]
      }
      event "Pectorales Bool": Value Change {
        n430 = event-data() -> ()  [unwired: 1 in, 6 out]
        n431 = Bundle By Name(cluster=cluster{"Color Box":u32, "Color Box 2":u32} {"Color Box"=12369084, "Color Box 2"=12369084}, "Color Box"=u32 16711680 ("Color Box 2")) -> (w971:cluster{"Color Box":u32, "Color Box 2":u32})
        n432 = Bundle By Name(cluster=cluster{"Color Box":u32, "Color Box 2":u32} {"Color Box"=12369084, "Color Box 2"=12369084}, "Color Box"=u32 12369084 ("Color Box 2")) -> (w967:cluster{"Color Box":u32, "Color Box 2":u32})
        n433 = Bundle By Name(cluster=w962, "Label"="Pectorales" ("Message")) -> (w961:T1)
        n434 = Insert Into Array(array=cluster{u32, u32}[] [] ("Colors [4]"), new element=w971) -> (w964:cluster{u32, u32}[])  [unwired: 1 in]
        n435 = Insert Into Array(array=cluster{u32, u32}[] [] ("Colors [4]"), new element=w967) -> (w965:cluster{u32, u32}[])  [unwired: 1 in]
        n436 = property on="Pectorales Bool" class="Bool"("Colors [4]"=w964) -> ()  [unwired: 2 in, 2 out]
        n437 = property on="Gluteos Bool" class="Bool"("Colors [4]"=w965) -> ()  [unwired: 2 in, 2 out]
        n438 = property on="Abdomen Bool" class="Bool"("Colors [4]"=w965) -> ()  [unwired: 2 in, 2 out]
        n439 = property on="Isquiotibiales Bool" class="Bool"("Colors [4]"=w965) -> ()  [unwired: 2 in, 2 out]
        n440 = property on="Cuadriceps Bool" class="Bool"("Colors [4]"=w965) -> ()  [unwired: 2 in, 2 out]
        n441 = property on="Trapecio Bool" class="Bool"("Colors [4]"=w965) -> ()  [unwired: 2 in, 2 out]
        n442 = property on="Lumbares Bool" class="Bool"("Colors [4]"=w965) -> ()  [unwired: 2 in, 2 out]
        n443 = property on="Dorsales Bool" class="Bool"("Colors [4]"=w965) -> ()  [unwired: 2 in, 2 out]
        n444 = property on="Opcional Bool" class="Bool"("Colors [4]"=w965) -> ()  [unwired: 2 in, 2 out]
        n445 = property on="Biceps Bool" class="Bool"("Colors [4]"=w965) -> ()  [unwired: 2 in, 2 out]
      }
      event "Biceps Bool": Value Change {
        n446 = event-data() -> ()  [unwired: 1 in, 6 out]
        n447 = Bundle By Name(cluster=cluster{"Color Box":u32, "Color Box 2":u32} {"Color Box"=12369084, "Color Box 2"=12369084}, "Color Box"=u32 16711680 ("Color Box 2")) -> (w985:cluster{"Color Box":u32, "Color Box 2":u32})
        n448 = Bundle By Name(cluster=cluster{"Color Box":u32, "Color Box 2":u32} {"Color Box"=12369084, "Color Box 2"=12369084}, "Color Box"=u32 12369084 ("Color Box 2")) -> (w981:cluster{"Color Box":u32, "Color Box 2":u32})
        n449 = Bundle By Name(cluster=w976, "Label"="Biceps" ("Message")) -> (w975:T1)
        n450 = Insert Into Array(array=cluster{u32, u32}[] [] ("Colors [4]"), new element=w985) -> (w978:cluster{u32, u32}[])  [unwired: 1 in]
        n451 = Insert Into Array(array=cluster{u32, u32}[] [] ("Colors [4]"), new element=w981) -> (w979:cluster{u32, u32}[])  [unwired: 1 in]
        n452 = property on="Biceps Bool" class="Bool"("Colors [4]"=w978) -> ()  [unwired: 2 in, 2 out]
        n453 = property on="Gluteos Bool" class="Bool"("Colors [4]"=w979) -> ()  [unwired: 2 in, 2 out]
        n454 = property on="Abdomen Bool" class="Bool"("Colors [4]"=w979) -> ()  [unwired: 2 in, 2 out]
        n455 = property on="Isquiotibiales Bool" class="Bool"("Colors [4]"=w979) -> ()  [unwired: 2 in, 2 out]
        n456 = property on="Cuadriceps Bool" class="Bool"("Colors [4]"=w979) -> ()  [unwired: 2 in, 2 out]
        n457 = property on="Trapecio Bool" class="Bool"("Colors [4]"=w979) -> ()  [unwired: 2 in, 2 out]
        n458 = property on="Lumbares Bool" class="Bool"("Colors [4]"=w979) -> ()  [unwired: 2 in, 2 out]
        n459 = property on="Dorsales Bool" class="Bool"("Colors [4]"=w979) -> ()  [unwired: 2 in, 2 out]
        n460 = property on="Opcional Bool" class="Bool"("Colors [4]"=w979) -> ()  [unwired: 2 in, 2 out]
        n461 = property on="Pectorales Bool" class="Bool"("Colors [4]"=w979) -> ()  [unwired: 2 in, 2 out]
      }
      event "Opcional Bool": Value Change {
        n462 = event-data() -> ()  [unwired: 1 in, 6 out]
        n463 = Bundle By Name(cluster=cluster{"Color Box":u32, "Color Box 2":u32} {"Color Box"=12369084, "Color Box 2"=12369084}, "Color Box"=u32 16711680 ("Color Box 2")) -> (w999:cluster{"Color Box":u32, "Color Box 2":u32})
        n464 = Bundle By Name(cluster=cluster{"Color Box":u32, "Color Box 2":u32} {"Color Box"=12369084, "Color Box 2"=12369084}, "Color Box"=u32 12369084 ("Color Box 2")) -> (w995:cluster{"Color Box":u32, "Color Box 2":u32})
        n465 = Bundle By Name(cluster=w990, "Label"="Opcional" ("Message")) -> (w989:T1)
        n466 = Insert Into Array(array=cluster{u32, u32}[] [] ("Colors [4]"), new element=w999) -> (w992:cluster{u32, u32}[])  [unwired: 1 in]
        n467 = Insert Into Array(array=cluster{u32, u32}[] [] ("Colors [4]"), new element=w995) -> (w993:cluster{u32, u32}[])  [unwired: 1 in]
        n468 = property on="Opcional Bool" class="Bool"("Colors [4]"=w992) -> ()  [unwired: 2 in, 2 out]
        n469 = property on="Gluteos Bool" class="Bool"("Colors [4]"=w993) -> ()  [unwired: 2 in, 2 out]
        n470 = property on="Abdomen Bool" class="Bool"("Colors [4]"=w993) -> ()  [unwired: 2 in, 2 out]
        n471 = property on="Isquiotibiales Bool" class="Bool"("Colors [4]"=w993) -> ()  [unwired: 2 in, 2 out]
        n472 = property on="Cuadriceps Bool" class="Bool"("Colors [4]"=w993) -> ()  [unwired: 2 in, 2 out]
        n473 = property on="Trapecio Bool" class="Bool"("Colors [4]"=w993) -> ()  [unwired: 2 in, 2 out]
        n474 = property on="Lumbares Bool" class="Bool"("Colors [4]"=w993) -> ()  [unwired: 2 in, 2 out]
        n475 = property on="Dorsales Bool" class="Bool"("Colors [4]"=w993) -> ()  [unwired: 2 in, 2 out]
        n476 = property on="Biceps Bool" class="Bool"("Colors [4]"=w993) -> ()  [unwired: 2 in, 2 out]
        n477 = property on="Pectorales Bool" class="Bool"("Colors [4]"=w993) -> ()  [unwired: 2 in, 2 out]
      }
      event "Add Button": Value Change {
        n478 = event-data() -> ()  [unwired: 1 in, 6 out]
        n479 = Unbundle By Name(w1006) -> ("Label"=w1005:string)
        n480 = case shown="\"Cuadriceps\"" w1005 {
          tunnel: [w1009 w1024 w1037 w1047 w1060 w1073 w1086 w1099 w1112 w1125 w1138 w1151] -> w1007
          tunnel: w1006 -> [w1020 w1033 w1046 w1059 w1072 w1085 w1098 w1111 w1124 w1137 w1150 w1151]
          tunnel: w1004 -> [w1011 w1023 w1036 w1048 w1062 w1075 w1087 w1101 w1114 w1127 w1140 _]
          tunnel: w1003 -> [w1010 w1022 w1035 w1049 w1061 w1074 w1088 w1100 w1113 w1126 w1139 _]
          frame "Cuadriceps" {
            n481 = Unbundle By Name(w1020) -> ("Cuadriceps"=w1012:i32)
            n482 = Greater Or Equal To 0?(x=w1012) -> (x >= 0?=w1017:bool)
            n483 = Less Or Equal?(x=w1012, y=100) -> (x <= y?=w1015:bool)
            n484 = Add(x=w1012, y=5) -> (x+y=w1019:i32)
            n485 = And(x=w1017, y=w1015) -> (x .and. y?=w1016:bool)
            n486 = Select(t=w1019, s=w1016, f=w1012) -> (s? t:f=w1013:i32)
            n487 = Bundle By Name(cluster=w1020, "Cuadriceps"=w1013, "Label"="Cuadriceps") -> (w1009:T1)
            n488 = Enqueue Element(queue=w1010, element=w1009, error in (no error)=w1011) -> ()  [unwired: 1 in, 3 out]
          }
          frame "Isquiotibiales" {
            n489 = Unbundle By Name(w1033) -> ("Isquiotibiales"=w1025:i32)
            n490 = Greater Or Equal To 0?(x=w1025) -> (x >= 0?=w1030:bool)
            n491 = Less Or Equal?(x=w1025, y=100) -> (x <= y?=w1028:bool)
            n492 = Add(x=w1025, y=5) -> (x+y=w1032:i32)
            n493 = And(x=w1030, y=w1028) -> (x .and. y?=w1029:bool)
            n494 = Select(t=w1032, s=w1029, f=w1025) -> (s? t:f=w1026:i32)
            n495 = Bundle By Name(cluster=w1033, "Isquiotibiales"=w1026, "Label"="Isquiotibiales") -> (w1024:T1)
            n496 = Enqueue Element(queue=w1022, element=w1024, error in (no error)=w1023) -> ()  [unwired: 1 in, 3 out]
          }
          frame "Gluteos" {
            n497 = Unbundle By Name(w1046) -> ("Gluteos"=w1038:i32)
            n498 = Greater Or Equal To 0?(x=w1038) -> (x >= 0?=w1043:bool)
            n499 = Less Or Equal?(x=w1038, y=100) -> (x <= y?=w1041:bool)
            n500 = Add(x=w1038, y=5) -> (x+y=w1045:i32)
            n501 = And(x=w1043, y=w1041) -> (x .and. y?=w1042:bool)
            n502 = Select(t=w1045, s=w1042, f=w1038) -> (s? t:f=w1039:i32)
            n503 = Bundle By Name(cluster=w1046, "Gluteos"=w1039, "Label"="Gluteos") -> (w1037:T1)
            n504 = Enqueue Element(queue=w1035, element=w1037, error in (no error)=w1036) -> ()  [unwired: 1 in, 3 out]
          }
          frame "Abdomen" {
            n505 = Unbundle By Name(w1059) -> ("Abdomen"=w1051:i32)
            n506 = Greater Or Equal To 0?(x=w1051) -> (x >= 0?=w1056:bool)
            n507 = Less Or Equal?(x=w1051, y=100) -> (x <= y?=w1054:bool)
            n508 = Add(x=w1051, y=5) -> (x+y=w1058:i32)
            n509 = And(x=w1056, y=w1054) -> (x .and. y?=w1055:bool)
            n510 = Select(t=w1058, s=w1055, f=w1051) -> (s? t:f=w1052:i32)
            n511 = Bundle By Name(cluster=w1059, "Abdomen"=w1052, "Label"="Abdomen") -> (w1047:T1)
            n512 = Enqueue Element(queue=w1049, element=w1047, error in (no error)=w1048) -> ()  [unwired: 1 in, 3 out]
          }
          frame "Lumbares" {
            n513 = Unbundle By Name(w1072) -> ("Lumbares"=w1064:i32)
            n514 = Greater Or Equal To 0?(x=w1064) -> (x >= 0?=w1069:bool)
            n515 = Less Or Equal?(x=w1064, y=100) -> (x <= y?=w1067:bool)
            n516 = Add(x=w1064, y=5) -> (x+y=w1071:i32)
            n517 = And(x=w1069, y=w1067) -> (x .and. y?=w1068:bool)
            n518 = Select(t=w1071, s=w1068, f=w1064) -> (s? t:f=w1065:i32)
            n519 = Bundle By Name(cluster=w1072, "Lumbares"=w1065, "Label"="Lumbares") -> (w1060:T1)
            n520 = Enqueue Element(queue=w1061, element=w1060, error in (no error)=w1062) -> ()  [unwired: 1 in, 3 out]
          }
          frame "Dorsales" {
            n521 = Unbundle By Name(w1085) -> ("Dorsales"=w1077:i32)
            n522 = Greater Or Equal To 0?(x=w1077) -> (x >= 0?=w1082:bool)
            n523 = Less Or Equal?(x=w1077, y=100) -> (x <= y?=w1080:bool)
            n524 = Add(x=w1077, y=5) -> (x+y=w1084:i32)
            n525 = And(x=w1082, y=w1080) -> (x .and. y?=w1081:bool)
            n526 = Select(t=w1084, s=w1081, f=w1077) -> (s? t:f=w1078:i32)
            n527 = Bundle By Name(cluster=w1085, "Dorsales"=w1078, "Label"="Dorsales") -> (w1073:T1)
            n528 = Enqueue Element(queue=w1074, element=w1073, error in (no error)=w1075) -> ()  [unwired: 1 in, 3 out]
          }
          frame "Trapecio" {
            n529 = Unbundle By Name(w1098) -> ("Trapecio"=w1090:i32)
            n530 = Greater Or Equal To 0?(x=w1090) -> (x >= 0?=w1095:bool)
            n531 = Less Or Equal?(x=w1090, y=100) -> (x <= y?=w1093:bool)
            n532 = Add(x=w1090, y=5) -> (x+y=w1097:i32)
            n533 = And(x=w1095, y=w1093) -> (x .and. y?=w1094:bool)
            n534 = Select(t=w1097, s=w1094, f=w1090) -> (s? t:f=w1091:i32)
            n535 = Bundle By Name(cluster=w1098, "Trapecio"=w1091, "Label"="Trapecio") -> (w1086:T1)
            n536 = Enqueue Element(queue=w1088, element=w1086, error in (no error)=w1087) -> ()  [unwired: 1 in, 3 out]
          }
          frame "Pectorales" {
            n537 = Unbundle By Name(w1111) -> ("Pectorales"=w1103:i32)
            n538 = Greater Or Equal To 0?(x=w1103) -> (x >= 0?=w1108:bool)
            n539 = Less Or Equal?(x=w1103, y=100) -> (x <= y?=w1106:bool)
            n540 = Add(x=w1103, y=5) -> (x+y=w1110:i32)
            n541 = And(x=w1108, y=w1106) -> (x .and. y?=w1107:bool)
            n542 = Select(t=w1110, s=w1107, f=w1103) -> (s? t:f=w1104:i32)
            n543 = Bundle By Name(cluster=w1111, "Pectorales"=w1104, "Label"="Pectorales") -> (w1099:T1)
            n544 = Enqueue Element(queue=w1100, element=w1099, error in (no error)=w1101) -> ()  [unwired: 1 in, 3 out]
          }
          frame "Biceps" {
            n545 = Unbundle By Name(w1124) -> ("Biceps"=w1116:i32)
            n546 = Greater Or Equal To 0?(x=w1116) -> (x >= 0?=w1121:bool)
            n547 = Less Or Equal?(x=w1116, y=100) -> (x <= y?=w1119:bool)
            n548 = Add(x=w1116, y=5) -> (x+y=w1123:i32)
            n549 = And(x=w1121, y=w1119) -> (x .and. y?=w1120:bool)
            n550 = Select(t=w1123, s=w1120, f=w1116) -> (s? t:f=w1117:i32)
            n551 = Bundle By Name(cluster=w1124, "Biceps"=w1117, "Label"="Biceps") -> (w1112:T1)
            n552 = Enqueue Element(queue=w1113, element=w1112, error in (no error)=w1114) -> ()  [unwired: 1 in, 3 out]
          }
          frame "Opcional" {
            n553 = Unbundle By Name(w1137) -> ("Opcional"=w1129:i32)
            n554 = Greater Or Equal To 0?(x=w1129) -> (x >= 0?=w1134:bool)
            n555 = Less Or Equal?(x=w1129, y=100) -> (x <= y?=w1132:bool)
            n556 = Add(x=w1129, y=5) -> (x+y=w1136:i32)
            n557 = And(x=w1134, y=w1132) -> (x .and. y?=w1133:bool)
            n558 = Select(t=w1136, s=w1133, f=w1129) -> (s? t:f=w1130:i32)
            n559 = Bundle By Name(cluster=w1137, "Opcional"=w1130, "Label"="Opcional") -> (w1125:T1)
            n560 = Enqueue Element(queue=w1126, element=w1125, error in (no error)=w1127) -> ()  [unwired: 1 in, 3 out]
          }
          frame "Master" {
            n561 = Unbundle By Name(w1150) -> ("Master"=w1142:i32)
            n562 = Greater Or Equal To 0?(x=w1142) -> (x >= 0?=w1147:bool)
            n563 = Less?(x=w1142, y=100) -> (x < y?=w1145:bool)
            n564 = Add(x=w1142, y=5) -> (x+y=w1149:i32)
            n565 = And(x=w1147, y=w1145) -> (x .and. y?=w1146:bool)
            n566 = Select(t=w1149, s=w1146, f=w1142) -> (s? t:f=w1143:i32)
            n567 = Bundle By Name(cluster=w1150, "Master"=w1143, "Label"="Master") -> (w1138:T1)
            n568 = Enqueue Element(queue=w1139, element=w1138, error in (no error)=w1140) -> ()  [unwired: 1 in, 3 out]
          }
          frame Default {
          }
        }
      }
      event "Remove Button": Value Change {
        n569 = event-data() -> ()  [unwired: 1 in, 6 out]
        n570 = Unbundle By Name(w1155) -> ("Label"=w1154:string)
        n571 = case shown="\"Cuadriceps\"" w1154 {
          tunnel: [w1157 w1168 w1177 w1187 w1197 w1207 w1218 w1227 w1237 w1247 w1257 w1267] -> w1156
          tunnel: w1155 -> [w1166 w1176 w1186 w1196 w1206 w1216 w1226 w1236 w1246 w1256 w1266 w1267]
          tunnel: w1153 -> [w1158 w1169 w1178 w1188 w1199 w1208 w1220 w1228 w1239 w1249 w1259 _]
          tunnel: w1152 -> [w1159 w1170 w1179 w1189 w1198 w1209 w1219 w1229 w1238 w1248 w1258 _]
          frame "Cuadriceps" {
            n572 = Unbundle By Name(w1166) -> ("Cuadriceps"=w1161:i32)
            n573 = Greater Than 0?(x=w1161) -> (x > 0?=w1163:bool)
            n574 = Subtract(x=w1161, y=5) -> (x-y=w1164:i32)
            n575 = Select(t=w1164, s=w1163, f=w1161) -> (s? t:f=w1162:i32)
            n576 = Bundle By Name(cluster=w1166, "Cuadriceps"=w1162, "Label"="Cuadriceps") -> (w1157:T1)
            n577 = Enqueue Element(queue=w1158, element=w1157, error in (no error)=w1159) -> ()  [unwired: 1 in, 3 out]
          }
          frame "Isquiotibiales" {
            n578 = Unbundle By Name(w1176) -> ("Isquiotibiales"=w1171:i32)
            n579 = Greater Than 0?(x=w1171) -> (x > 0?=w1173:bool)
            n580 = Subtract(x=w1171, y=5) -> (x-y=w1174:i32)
            n581 = Select(t=w1174, s=w1173, f=w1171) -> (s? t:f=w1172:i32)
            n582 = Bundle By Name(cluster=w1176, "Isquiotibiales"=w1172, "Label"="Isquiotibiales") -> (w1168:T1)
            n583 = Enqueue Element(queue=w1169, element=w1168, error in (no error)=w1170) -> ()  [unwired: 1 in, 3 out]
          }
          frame "Gluteos" {
            n584 = Unbundle By Name(w1186) -> ("Gluteos"=w1181:i32)
            n585 = Greater Than 0?(x=w1181) -> (x > 0?=w1183:bool)
            n586 = Subtract(x=w1181, y=5) -> (x-y=w1184:i32)
            n587 = Select(t=w1184, s=w1183, f=w1181) -> (s? t:f=w1182:i32)
            n588 = Bundle By Name(cluster=w1186, "Gluteos"=w1182, "Label"="Gluteos") -> (w1177:T1)
            n589 = Enqueue Element(queue=w1178, element=w1177, error in (no error)=w1179) -> ()  [unwired: 1 in, 3 out]
          }
          frame "Abdomen" {
            n590 = Unbundle By Name(w1196) -> ("Abdomen"=w1191:i32)
            n591 = Greater Than 0?(x=w1191) -> (x > 0?=w1193:bool)
            n592 = Subtract(x=w1191, y=5) -> (x-y=w1194:i32)
            n593 = Select(t=w1194, s=w1193, f=w1191) -> (s? t:f=w1192:i32)
            n594 = Bundle By Name(cluster=w1196, "Abdomen"=w1192, "Label"="Abdomen") -> (w1187:T1)
            n595 = Enqueue Element(queue=w1188, element=w1187, error in (no error)=w1189) -> ()  [unwired: 1 in, 3 out]
          }
          frame "Lumbares" {
            n596 = Unbundle By Name(w1206) -> ("Lumbares"=w1201:i32)
            n597 = Greater Than 0?(x=w1201) -> (x > 0?=w1203:bool)
            n598 = Subtract(x=w1201, y=5) -> (x-y=w1204:i32)
            n599 = Select(t=w1204, s=w1203, f=w1201) -> (s? t:f=w1202:i32)
            n600 = Bundle By Name(cluster=w1206, "Lumbares"=w1202, "Label"="Lumbares") -> (w1197:T1)
            n601 = Enqueue Element(queue=w1199, element=w1197, error in (no error)=w1198) -> ()  [unwired: 1 in, 3 out]
          }
          frame "Dorsales" {
            n602 = Unbundle By Name(w1216) -> ("Dorsales"=w1211:i32)
            n603 = Greater Than 0?(x=w1211) -> (x > 0?=w1213:bool)
            n604 = Subtract(x=w1211, y=5) -> (x-y=w1214:i32)
            n605 = Select(t=w1214, s=w1213, f=w1211) -> (s? t:f=w1212:i32)
            n606 = Bundle By Name(cluster=w1216, "Dorsales"=w1212, "Label"="Dorsales") -> (w1207:T1)
            n607 = Enqueue Element(queue=w1208, element=w1207, error in (no error)=w1209) -> ()  [unwired: 1 in, 3 out]
          }
          frame "Trapecio" {
            n608 = Unbundle By Name(w1226) -> ("Trapecio"=w1221:i32)
            n609 = Greater Than 0?(x=w1221) -> (x > 0?=w1223:bool)
            n610 = Subtract(x=w1221, y=5) -> (x-y=w1224:i32)
            n611 = Select(t=w1224, s=w1223, f=w1221) -> (s? t:f=w1222:i32)
            n612 = Bundle By Name(cluster=w1226, "Trapecio"=w1222, "Label"="Trapecio") -> (w1218:T1)
            n613 = Enqueue Element(queue=w1220, element=w1218, error in (no error)=w1219) -> ()  [unwired: 1 in, 3 out]
          }
          frame "Pectorales" {
            n614 = Unbundle By Name(w1236) -> ("Pectorales"=w1231:i32)
            n615 = Greater Than 0?(x=w1231) -> (x > 0?=w1233:bool)
            n616 = Subtract(x=w1231, y=5) -> (x-y=w1234:i32)
            n617 = Select(t=w1234, s=w1233, f=w1231) -> (s? t:f=w1232:i32)
            n618 = Bundle By Name(cluster=w1236, "Pectorales"=w1232, "Label"="Pectorales") -> (w1227:T1)
            n619 = Enqueue Element(queue=w1228, element=w1227, error in (no error)=w1229) -> ()  [unwired: 1 in, 3 out]
          }
          frame "Biceps" {
            n620 = Unbundle By Name(w1246) -> ("Biceps"=w1241:i32)
            n621 = Greater Than 0?(x=w1241) -> (x > 0?=w1243:bool)
            n622 = Subtract(x=w1241, y=5) -> (x-y=w1244:i32)
            n623 = Select(t=w1244, s=w1243, f=w1241) -> (s? t:f=w1242:i32)
            n624 = Bundle By Name(cluster=w1246, "Biceps"=w1242, "Label"="Biceps") -> (w1237:T1)
            n625 = Enqueue Element(queue=w1239, element=w1237, error in (no error)=w1238) -> ()  [unwired: 1 in, 3 out]
          }
          frame "Opcional" {
            n626 = Unbundle By Name(w1256) -> ("Opcional"=w1251:i32)
            n627 = Greater Than 0?(x=w1251) -> (x > 0?=w1253:bool)
            n628 = Subtract(x=w1251, y=5) -> (x-y=w1254:i32)
            n629 = Select(t=w1254, s=w1253, f=w1251) -> (s? t:f=w1252:i32)
            n630 = Bundle By Name(cluster=w1256, "Opcional"=w1252, "Label"="Opcional") -> (w1247:T1)
            n631 = Enqueue Element(queue=w1249, element=w1247, error in (no error)=w1248) -> ()  [unwired: 1 in, 3 out]
          }
          frame "Master" {
            n632 = Unbundle By Name(w1266) -> ("Master"=w1261:i32)
            n633 = Greater Than 0?(x=w1261) -> (x > 0?=w1263:bool)
            n634 = Subtract(x=w1261, y=5) -> (x-y=w1264:i32)
            n635 = Select(t=w1264, s=w1263, f=w1261) -> (s? t:f=w1262:i32)
            n636 = Bundle By Name(cluster=w1266, "Master"=w1262, "Label"="Master") -> (w1257:T1)
            n637 = Enqueue Element(queue=w1259, element=w1257, error in (no error)=w1258) -> ()  [unwired: 1 in, 3 out]
          }
          frame Default {
          }
        }
      }
      event "Slider": Value Change {
        n638 = event-data() -> ()  [unwired: 1 in, 6 out]
        n639 = Unbundle By Name(w1272) -> ("Label"=w1270:string)
        n640 = case shown="\"Cuadriceps\"" w1270 {
          tunnel: [w1274 w1280 w1286 w1292 w1298 w1304 w1310 w1316 w1322 w1328 w1334 w1340] -> w1273
          tunnel: w1272 -> [w1279 w1285 w1291 w1297 w1303 w1309 w1315 w1321 w1327 w1333 w1339 w1340]
          tunnel: "Slider" -> [w1278 w1284 w1290 w1296 w1302 w1308 w1314 w1320 w1326 w1332 w1338 _]
          tunnel: w1269 -> [w1275 w1282 w1288 w1294 w1299 w1306 w1312 w1318 w1324 w1330 w1336 _]
          tunnel: w1268 -> [w1276 w1281 w1287 w1293 w1300 w1305 w1311 w1317 w1323 w1329 w1335 _]
          frame "Cuadriceps" {
            n641 = Bundle By Name(cluster=w1279, "Cuadriceps"=w1278, "Label"="Cuadriceps") -> (w1274:T1)
            n642 = Enqueue Element(queue=w1276, element=w1274, error in (no error)=w1275) -> ()  [unwired: 1 in, 3 out]
          }
          frame "Isquiotibiales" {
            n643 = Bundle By Name(cluster=w1285, "Isquiotibiales"=w1284, "Label"="Isquiotibiales") -> (w1280:T1)
            n644 = Enqueue Element(queue=w1281, element=w1280, error in (no error)=w1282) -> ()  [unwired: 1 in, 3 out]
          }
          frame "Gluteos" {
            n645 = Bundle By Name(cluster=w1291, "Gluteos"=w1290, "Label"="Gluteos") -> (w1286:T1)
            n646 = Enqueue Element(queue=w1287, element=w1286, error in (no error)=w1288) -> ()  [unwired: 1 in, 3 out]
          }
          frame "Abdomen" {
            n647 = Bundle By Name(cluster=w1297, "Abdomen"=w1296, "Label"="Abdomen") -> (w1292:T1)
            n648 = Enqueue Element(queue=w1293, element=w1292, error in (no error)=w1294) -> ()  [unwired: 1 in, 3 out]
          }
          frame "Lumbares" {
            n649 = Bundle By Name(cluster=w1303, "Lumbares"=w1302, "Label"="Lumbares") -> (w1298:T1)
            n650 = Enqueue Element(queue=w1300, element=w1298, error in (no error)=w1299) -> ()  [unwired: 1 in, 3 out]
          }
          frame "Dorsales" {
            n651 = Bundle By Name(cluster=w1309, "Dorsales"=w1308, "Label"="Dorsales") -> (w1304:T1)
            n652 = Enqueue Element(queue=w1305, element=w1304, error in (no error)=w1306) -> ()  [unwired: 1 in, 3 out]
          }
          frame "Trapecio" {
            n653 = Bundle By Name(cluster=w1315, "Trapecio"=w1314, "Label"="Trapecio") -> (w1310:T1)
            n654 = Enqueue Element(queue=w1311, element=w1310, error in (no error)=w1312) -> ()  [unwired: 1 in, 3 out]
          }
          frame "Pectorales" {
            n655 = Bundle By Name(cluster=w1321, "Pectorales"=w1320, "Label"="Pectorales") -> (w1316:T1)
            n656 = Enqueue Element(queue=w1317, element=w1316, error in (no error)=w1318) -> ()  [unwired: 1 in, 3 out]
          }
          frame "Biceps" {
            n657 = Bundle By Name(cluster=w1327, "Biceps"=w1326, "Label"="Biceps") -> (w1322:T1)
            n658 = Enqueue Element(queue=w1323, element=w1322, error in (no error)=w1324) -> ()  [unwired: 1 in, 3 out]
          }
          frame "Opcional" {
            n659 = Bundle By Name(cluster=w1333, "Opcional"=w1332, "Label"="Opcional") -> (w1328:T1)
            n660 = Enqueue Element(queue=w1329, element=w1328, error in (no error)=w1330) -> ()  [unwired: 1 in, 3 out]
          }
          frame "Master" {
            n661 = Bundle By Name(cluster=w1339, "Master"=w1338, "Label"="Master") -> (w1334:T1)
            n662 = Enqueue Element(queue=w1335, element=w1334, error in (no error)=w1336) -> ()  [unwired: 1 in, 3 out]
          }
          frame Default {
          }
        }
      }
      event "Stop": Value Change {
        n663 = event-data() -> ()  [unwired: 1 in, 6 out]
      }
      event "Back": Value Change {
        n664 = event-data() -> ()  [unwired: 1 in, 6 out]
        n665 = Bundle By Name(cluster=w1345, "Label"="Back" ("Message")) -> (w1343:T1)
      }
      event "Master": Value Change {
        n666 = event-data() -> ()  [unwired: 1 in, 6 out]
        n667 = property on="Master" class="Bool (strict)"() -> ("Colors [4]"=w1348:cluster{u32, u32}[])  [unwired: 2 in, 2 out]
        n668 = Index Array(array=w1348) -> (element=w1351:cluster{u32, u32})  [unwired: 1 in]
        n669 = Bundle By Name(cluster=w1356, "Label"="Master" ("Message")) -> (w1354:T1)
        n670 = Unbundle(w1351) -> (w1350:u32, w1349:u32)
        n671 = case shown="True" "Master" {
          tunnel: [u32 16711680 ("Boolean Text.Text Colors:Text Color") u32 16448250 ("Boolean Text.Text Colors:Text Color")] -> w1352
          tunnel: w1350 -> [_ w1365]
          tunnel: w1349 -> [w1363 _]
          tunnel: w1348 -> [w1361 w1367]
          tunnel: [w1358 w1368] -> w1347
          frame False {
            n672 = Bundle("Boolean Text.Text Colors:Text Color"=u32 13816530, w1363) -> (w1360:T2)  [unwired: 1 in]
            n673 = Replace Array Subset(array=w1361, new element=w1360, index=0) -> (w1358:cluster{u32, u32}[])
          }
          frame True {
            n674 = Bundle(w1365, "Boolean Text.Text Colors:Text Color"=u32 16711680) -> (w1370:T3)  [unwired: 1 in]
            n675 = Replace Array Subset(array=w1367, new element=w1370, index=0) -> (w1368:cluster{u32, u32}[])
          }
        }
        n676 = property on="Master" class="Bool (strict)"("BoolText.TextColor"=w1352) -> ()  [unwired: 2 in, 2 out]
        n677 = property on="Master" class="Bool (strict)"("Colors [4]"=w1347) -> ()  [unwired: 2 in, 2 out]
      }
      event "Help": Value Change {
        n678 = event-data() -> ()  [unwired: 1 in, 6 out]
        n679 = call "Help.vi"() -> ()  [unwired: 11 in, 1 out]
      }
      event "Impulso": Value Change {
        n680 = event-data() -> ()  [unwired: 1 in, 6 out]
        n681 = call "Impulso.vi"() -> ("Parametros"=w1388:cluster{i32, i32, i32, i32, i32, dbl})  [unwired: 2 in]
        n682 = Unbundle(w1388) -> (w1381:i32, w1374:i32, w1378:dbl)  [unwired: 3 out]
        n683 = Bundle By Name(cluster=w1389, "Label"="Frecuencia" ("Message"), "Frecuencia"=w1381) -> (w1380:T1)
        n684 = Enqueue Element(queue=w1387, element=w1380, error in (no error)=w1386) -> (queue out=w1384:refnum<queue>, error out=w1385:errorcluster)  [unwired: 1 in, 1 out]
        n685 = Bundle By Name(cluster=w1380, "Label"="Ganancia", "Ganancia"=w1378) -> (w1377:T1)
        n686 = Enqueue Element(queue=w1384, element=w1377, error in (no error)=w1385) -> (queue out=w1382:refnum<queue>, error out=w1383:errorcluster)  [unwired: 1 in, 1 out]
        n687 = Bundle By Name(cluster=w1377, "Label"="Impulso", "Impulso"=w1374) -> (w1375:T1)
        n688 = Enqueue Element(queue=w1382, element=w1375, error in (no error)=w1383) -> ()  [unwired: 1 in, 3 out]
      }
      event "Reset": Value Change {
        n689 = event-data() -> ()  [unwired: 1 in, 6 out]
        n690 = Bundle By Name(cluster=w1441, "Label"="Cuadriceps" ("Message"), "Cuadriceps"=0) -> (w1434:T1)
        n691 = Enqueue Element(queue=w1440, element=w1434, error in (no error)=w1439) -> (queue out=w1437:refnum<queue>, error out=w1438:errorcluster)  [unwired: 1 in, 1 out]
        n692 = Bundle By Name(cluster=w1434, "Label"="Isquiotibiales", "Isquiotibiales"=0) -> (w1432:T1)
        n693 = Enqueue Element(queue=w1437, element=w1432, error in (no error)=w1438) -> (queue out=w1435:refnum<queue>, error out=w1436:errorcluster)  [unwired: 1 in, 1 out]
        n694 = Bundle By Name(cluster=w1432, "Label"="Gluteos", "Gluteos"=0) -> (w1423:T1)
        n695 = Enqueue Element(queue=w1435, element=w1423, error in (no error)=w1436) -> (queue out=w1426:refnum<queue>, error out=w1427:errorcluster)  [unwired: 1 in, 1 out]
        n696 = Bundle By Name(cluster=w1423, "Label"="Abdomen", "Abdomen"=0) -> (w1420:T1)
        n697 = Enqueue Element(queue=w1426, element=w1420, error in (no error)=w1427) -> (queue out=w1424:refnum<queue>, error out=w1425:errorcluster)  [unwired: 1 in, 1 out]
        n698 = Bundle By Name(cluster=w1420, "Label"="Lumbares", "Lumbares"=0) -> (w1417:T1)
        n699 = Enqueue Element(queue=w1424, element=w1417, error in (no error)=w1425) -> (queue out=w1413:refnum<queue>, error out=w1414:errorcluster)  [unwired: 1 in, 1 out]
        n700 = Bundle By Name(cluster=w1417, "Label"="Dorsales", "Dorsales"=0) -> (w1410:T1)
        n701 = Bundle By Name(cluster=w1410, "Label"="Trapecio", "Trapecio"=0) -> (w1407:T1)
        n702 = Enqueue Element(queue=w1413, element=w1410, error in (no error)=w1414) -> (queue out=w1411:refnum<queue>, error out=w1412:errorcluster)  [unwired: 1 in, 1 out]
        n703 = Enqueue Element(queue=w1411, element=w1407, error in (no error)=w1412) -> (queue out=w1404:refnum<queue>, error out=w1403:errorcluster)  [unwired: 1 in, 1 out]
        n704 = Bundle By Name(cluster=w1407, "Label"="Pectorales", "Pectorales"=0) -> (w1402:T1)
        n705 = Bundle By Name(cluster=w1402, "Label"="Biceps", "Biceps"=0) -> (w1397:T1)
        n706 = Enqueue Element(queue=w1404, element=w1402, error in (no error)=w1403) -> (queue out=w1398:refnum<queue>, error out=w1399:errorcluster)  [unwired: 1 in, 1 out]
        n707 = Enqueue Element(queue=w1398, element=w1397, error in (no error)=w1399) -> (queue out=w1393:refnum<queue>, error out=w1394:errorcluster)  [unwired: 1 in, 1 out]
        n708 = Bundle By Name(cluster=w1397, "Label"="Opcional", "Opcional"=0) -> (w1392:T1)
        n709 = Enqueue Element(queue=w1393, element=w1392, error in (no error)=w1394) -> ()  [unwired: 1 in, 3 out]
      }
      event "Start": Value Change {
        n710 = event-data() -> ()  [unwired: 1 in, 6 out]
        n711 = Bundle By Name(cluster=w1446, "Label"="Start" ("Message")) -> (w1445:T1)
        "Boolean" <- "Start"
      }
    }
  }
  n712 = VISA Close(VISA resource name=w8, error in (no error)=w9) -> (error out=→"error out 2":errorcluster)
  n713 = Release Queue(queue=w2) -> ()  [unwired: 2 in, 3 out]
  "error out" <- "error in (no error)"
